vi "RG TAS v4b.vi"() -> ()   [LabVIEW 2015]
uses:
  <vilib>/Analysis/2dsp.llb/Decimate (single shot, DBL).vi
  <vilib>/DAQmx/read.llb/DAQmx Read (Analog Wfm 1Chan NSamp).vi
  Chaz TAS - DR/Sub VIs/Mono/global_Test.vi
  <vilib>/Instr/_visa.llb/VISA Configure Serial Port (Instr).vi
  Sub VIs/global tas.vi
  <vilib>/DAQmx/miscellaneous.llb/DAQmx Fill In Error Info.vi
  <vilib>/Utility/file.llb/Write To Spreadsheet File (DBL).vi
  <vilib>/Waveform/WDTOps.llb/WDT Index Channel DBL.vi
  Program Files/National Instruments/LabVIEW 2014/instr.lib/Tektronix DPO MSO 2000 4000 Series/Tektronix DPO MSO 2000 4000 Series.lvlib
  <vilib>/Analysis/NI_AALPro.lvlib
panel:
  in  "Inspect Traces":bool
  out "DAQ Loop":i32
  out "Scope Error Counter":i32
  out "Scope time axis":dbl[](array[numeric])
  in  "Stop acquisition":bool
  out "Grating":i32
  in  "2b - Spectrum":bool
  in  "2a - Kinetic":bool
  in  "Stop":bool
  out "Btrace Readout Counter":i32=2
  in  "Stop Btrace Measurement":bool
  out "Readout Counter":i32=2
  in  "Stop Measurement":bool
  in  "Calculate Output Method":T1(ring)
  in  "Parameters":T2(tab)
  in  "Shutter flow control":u16(ring) items=["None"=0, "XON/XOFF"=1, "RTS/CTS"=2, "DTR/DSR"=4]
  in  "Shutter stop bits":u16(ring)=10 items=["1.0"=10, "1.5"=15, "2.0"=20]
  in  "Shutter parity":u16(ring) items=["None", "Odd", "Even", "Mark", "Space"]
  in  "Shutter data bits":u16=8 min=5 max=8 step=1
  in  "Shutter VISA resource name":refnum<visa-resource-name>="COM1"
  in  "Shutter baud rate":u32=9600
  in  "Shutter open string":string="+100 10\n"
  in  "1 - Move Shutter":bool
  in  "3 - Move mono":bool
  out "Current wavelength (Oriel)":dbl format="%#_13g"
  in  "Monochromator Type":bool
  out "Start Wavelength":dbl min=0.0 format="%.3f"
  out "End Wavelength":dbl=100.0 min=0.0 format="%.3f"
  out "Interval Wavelength":dbl=10.0 min=0.0 format="%.3f"
  out "Current Wavelength (PTI)":dbl=300.0 min=300.0 max=2000.0 step=1.0
  in  "Is IR":bool caption="Grating"
  in  "Mono VISA name":refnum<visa-resource-name>
  in  "Mono 2 VISA name":refnum<visa-resource-name>
  out "DAQ dt":dbl=5e-06
  in  "DAQ End Time (s)":dbl=0.05
  in  "DAQ rate":i32=1250000
  in  "DAQ Trigger Level (V)":dbl=0.2
  out "DAQ Number of Samples":dbl=10000.0
  in  "DAQ average number of points":dbl=1.0
  out "DAQ final number of points":dbl
  in  "DAQ Input Channel":tag="Dev1/ai0"
  in  "100% Reflectance Standard (V)":dbl=1.0
  in  "DAQ Card":enum16{"USB-6211", "USB-6251"}(ring)=enum."USB-6251"
  in  "DAQ Input Config":i32(ring)=10106 items=["default"=-1, "RSE"=10083, "NRSE"=10078, "Differential"=10106, "Pseudodifferential"=12529]
  in  "Record Length":u32(ring)=10 items=["1000 points"=1, "10k points"=10, "100k points"=100, "1M points"=1000, "5M points"=5000, "10M points"=10000]
  in  "Acquisition Type":u16(ring)=2 items=["Sample", "Peak Detect", "Hi Res", "Envelope", "Average"]
  in  "Scope average\nnumber of points":dbl=1.0
  in  "Averages on scope":i32=1
  in  "Using TDS Scope?":bool
  in  "CH2 Impedance":u16(ring) items=["1M", "75", "50"]
  in  "CH1 Impedance":u16(ring)=2 items=["1M", "75", "50"]
  in  "Scope VISA resource name":refnum<visa-resource-name>="USB0::0x0699::0x0410::C022077::INSTR"
  in  "Scope Timeout (ms)":u32=30000
  in  "Channel TAS (0: Channel 1)":u16(ring) caption="Channel TAS" items=["Channel 1", "Channel 2", "Channel 3", "Channel 4", "Math", "Reference A", "Reference B", "Reference C", "Reference D"]
  in  "Channel TPC (0: Channel 1)":u16(ring)=1 caption="Channel TPC" items=["Channel 1", "Channel 2", "Channel 3", "Channel 4", "Math", "Reference A", "Reference B", "Reference C", "Reference D"]
  in  "Scope Timebase":dbl=0.0004 format="%^#_3e"
  in  "Trigger Source":u16(ring)=1 items=["Channel 1", "Channel 2", "Channel 3", "Channel 4", "AC Line", "Aux", "Digital Channel 0", "Digital Channel 1", "Digital Channel 2", "Digital Channel 3", "Digital Channel 4", "Digital Channel 5", "Digital Channel 6", "Digital Channel 7", "Digital Channel 8", "Digital Channel 9", "Digital Channel 10", "Digital Channel 11", "Digital Channel 12", "Digital Channel 13", "Digital Channel 14", "Digital Channel 15", "RF"]
  out "Final number of\nscope points":dbl=10000.0
  in  "Vertical Coupling TAS (1: DC)":u16(ring)=1 caption="Vertical Coupling TAS" items=["AC", "DC", "Ground"]
  in  "Probe Attenuation TAS (10.0)":dbl=1.0 caption="Probe Attenuation TAS"
  in  "Bandwidth CHTAS (0: FULL)":i32(ring) caption="Bandwidth CH TAS" items=["FULL", "250 MHz", "150 MHz", "20 MHz"]
  in  "Vertical Offset CH TAS (0.0 divs)":dbl=0.4 caption="Vertical Offset CH TAS (in V)"
  in  "Vertical Range CH TAS (10.0 V)":dbl=0.2 caption="Vertical Range CH TAS"
  in  "Trigger Level (V)":dbl=0.25
  in  "Vertical Coupling TPC (1: DC)":u16(ring)=1 caption="Vertical Coupling TPC" items=["AC", "DC", "Ground"]
  in  "Probe Attenuation TPC (1.0)":dbl=1.0 caption="Probe Attenuation TPC"
  in  "Vertical Range TPC (10.0 V)":dbl=0.2 caption="Vertical Range TPC"
  in  "Bandwidth CH TPC (0: FULL)":i32(ring) caption="Bandwidth CH TPC" items=["FULL", "250 MHz", "150 MHz", "20 MHz"]
  in  "Vertical Offset CH TPC (0.0 divs)":dbl caption="Vertical Offset CH TPC (in V)"
  in  "TPC Multiplication factor":dbl=1.0
  out "Number of scope readouts":i32
  in  "Scope Channel Read":bool
  in  "LED on (s)":dbl
  in  "LED off (s)":dbl
  in  "PIA Mode":bool
  in  "LEDs (constant irrad.)":bool caption="LEDs"
  in  "DAQ LED line":string="Dev1/port1/line0"
  in  "Control LEDs?":bool
  out "Scope pretrigger points":dbl=1000.0
  out "Scope CH1 DOD data (A-B final)":waveform(dbl)(graph)
  out "Scope CH1 DOD data (A final)":waveform(dbl)(graph)={"t0"=timestamp(-4.0000000000040004e-05 s since 1904-01-01), "dt"=4.0000000000000003e-07, "Y"=array[10000 elements]}
  out "Scope CH2 data (final)":waveform(dbl)(graph)={"t0"=timestamp(-4.0000000000040004e-05 s since 1904-01-01), "dt"=4.0000000000000003e-07, "Y"=array[10000 elements]}
  out "DAQ DOD data (final)":waveform(dbl)(graph)={"t0"=timestamp(0 s since 1904-01-01), "dt"=5e-06, "Y"=array[10000 elements]}
  out "B trace (Channel1)":waveform(dbl)(graph)
  in  "Amplification Factor":dbl=400.0
  out "Background level (on Amp)":dbl=30.577247161746392
  out "Background level (V)":dbl=0.08993307988748939
  in  "Trace B ?":bool
  out "Folder Created":bool
  in  "Sample Name":string="Sample"
  in  "TAS2014  Path":path=path "D:/Solar Fuels Data" caption="Folder"
  out "Path to Files":path=path "D:/Solar Fuels Data/Sample"
  out "Scope Average Channel2":waveform(dbl)(graph)={"t0"=timestamp(-4.0000000000040004e-05 s since 1904-01-01), "dt"=4.0000000000000003e-07, "Y"=array[10000 elements]}
  out "Scope Average Channel1":waveform(dbl)(graph)={"t0"=timestamp(-4.0000000000040004e-05 s since 1904-01-01), "dt"=4.0000000000000003e-07, "Y"=array[10000 elements]}
  out "DAQ Average Data":waveform(dbl)(graph)={"t0"=timestamp(0 s since 1904-01-01), "dt"=5e-06, "Y"=array[10000 elements]}
  in  "Number of Averages":i32=2
  out "DAQ Live Data":waveform(dbl)(graph)={"t0"=timestamp(0 s since 1904-01-01), "dt"=4.999999999999959e-06, "Y"=array[10000 elements]}
  # "Acquisition"
  # "Format: +100\\s20\\n OR \\F3\\002\\C1"
  # "Set COM ports for PTI\nmonochromators. If there\nis only 1 monochromator\npresent, leave Mono 2\nVISA name empty."
  # "DAQ Controls"
  # "DAQ Indicators"
  # "(Max = 250k/1.25M for\n6211/6251 DAQ cards)"
  # "Default is differential (connected ports are 15 and 16 on DAQ card).\n* For CH-TAS, input config should be RSE."
  # "Recommended Parameters for Different Scope Models"
  # "DPO3012"
  # "Record Length = 10k\nScope average number of points = 1"
  # "Acquisition Type = Hi Res\nAverages on scope = 1"
  # "DPO2012B"
  # "Record Length = 1M\nScope average number of points = 100"
  # "Acquisition Type = Average\nAverages on scope = 4"
  # "TDS3012C"
  # "Record Length = 10k\nScope average number of points = 1"
  # "Acquisition Type = Sample\nAverages on scope = 1"
  # "Channel 1"
  # "Channel 2"
  # "* For DPO2012B, impedance must be 1M for both channels!"
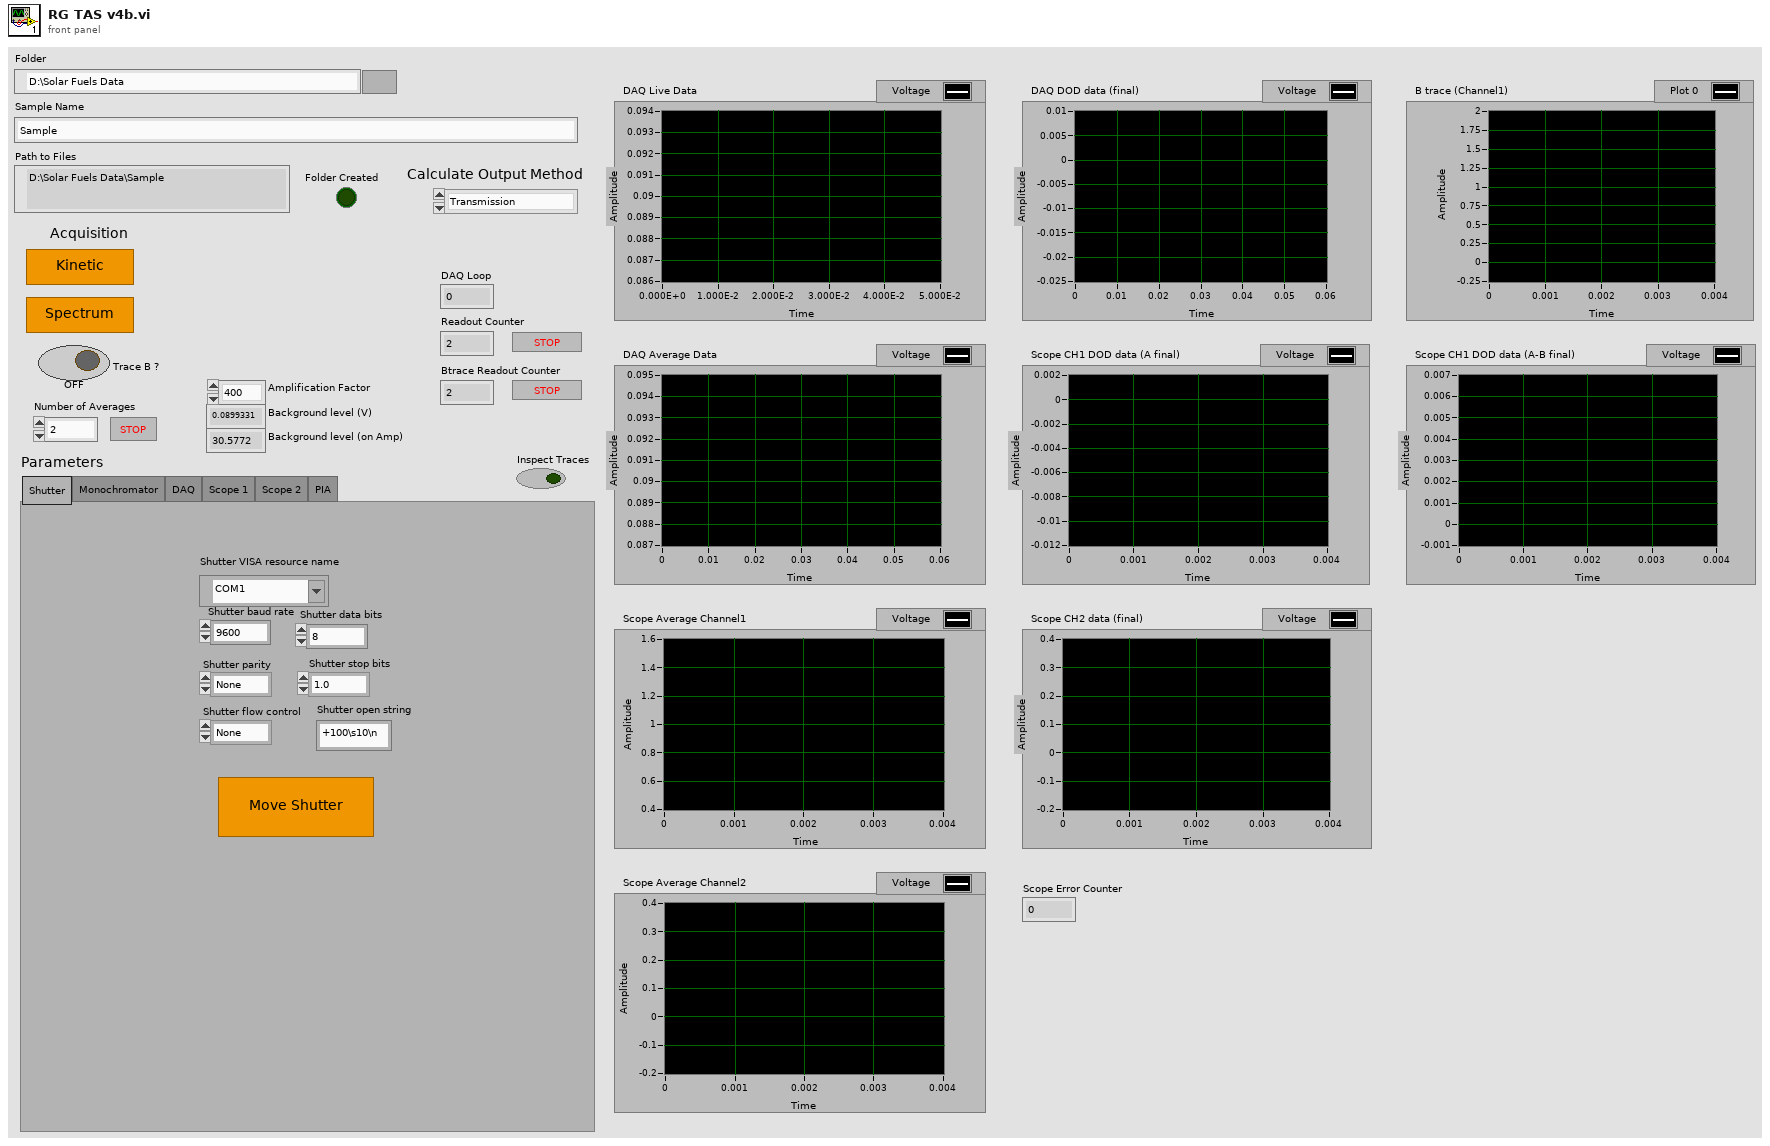
[diagram p1: front panel]
types:
  T1 = enum16{"Transmission", "Reflectance", "Kubelka-Munk"}
  T2 = enum32{"Shutter", "Monochromator", "DAQ", "Scope 1", "Scope 2", "PIA"}
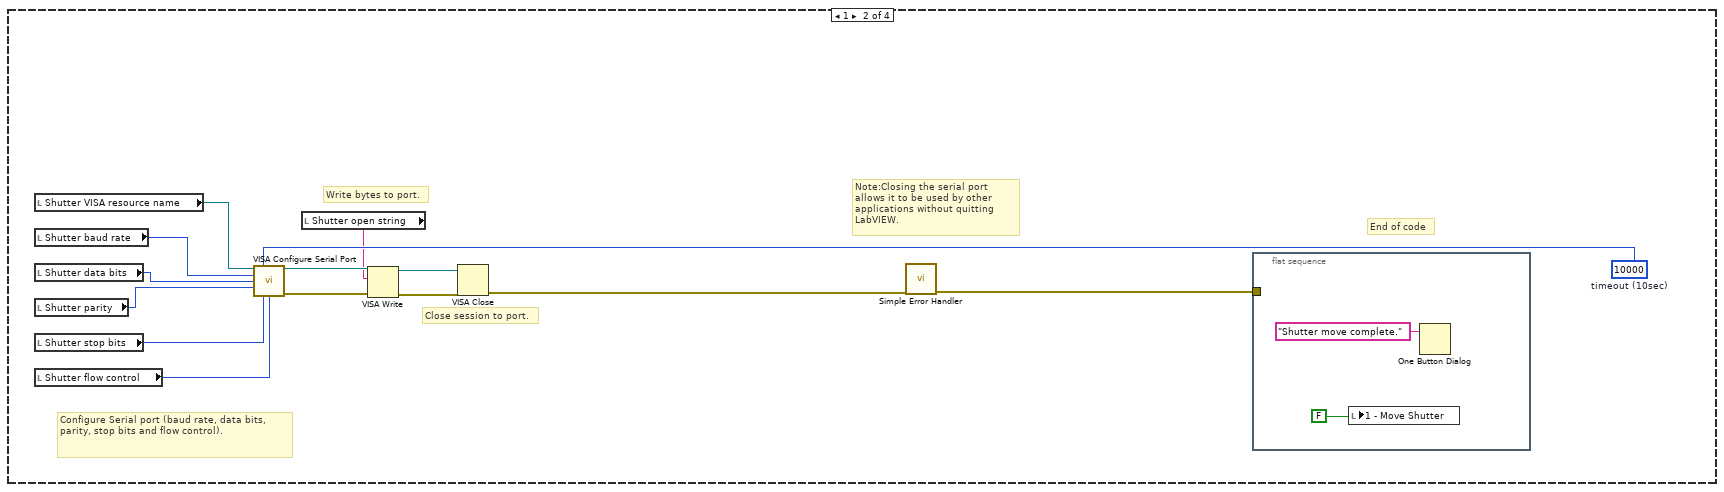
[diagram p4: hidden frame]
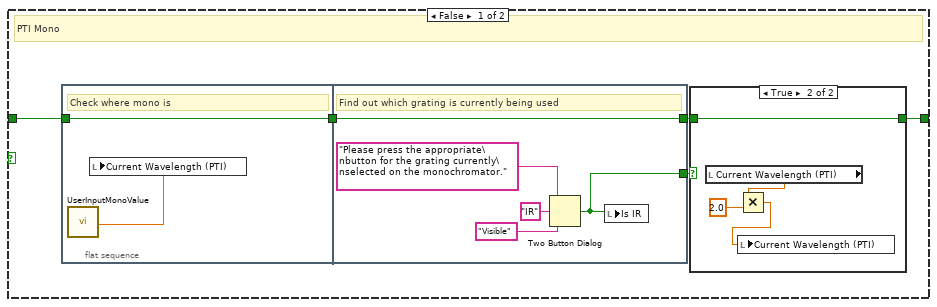
[diagram p5: hidden frame]
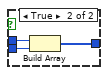
[diagram p8: hidden frame]
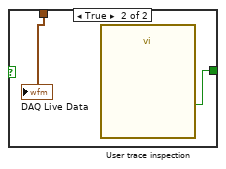
[diagram p9: hidden frame]
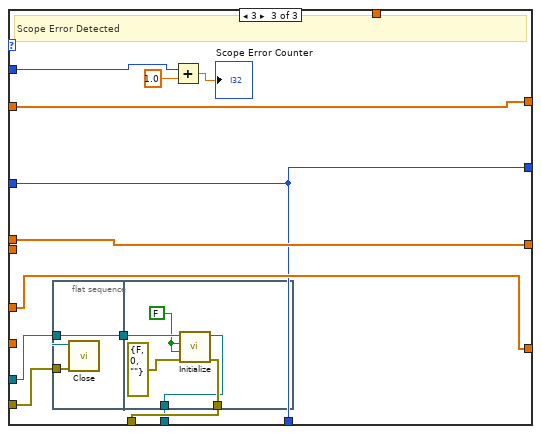
[diagram p11: hidden frame]
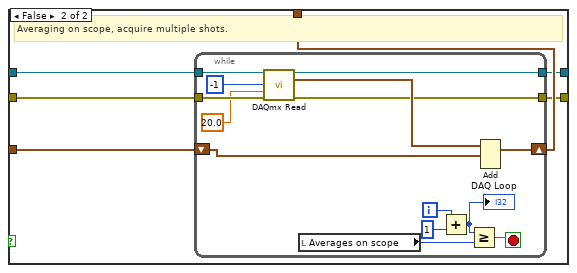
[diagram p13: hidden frame]
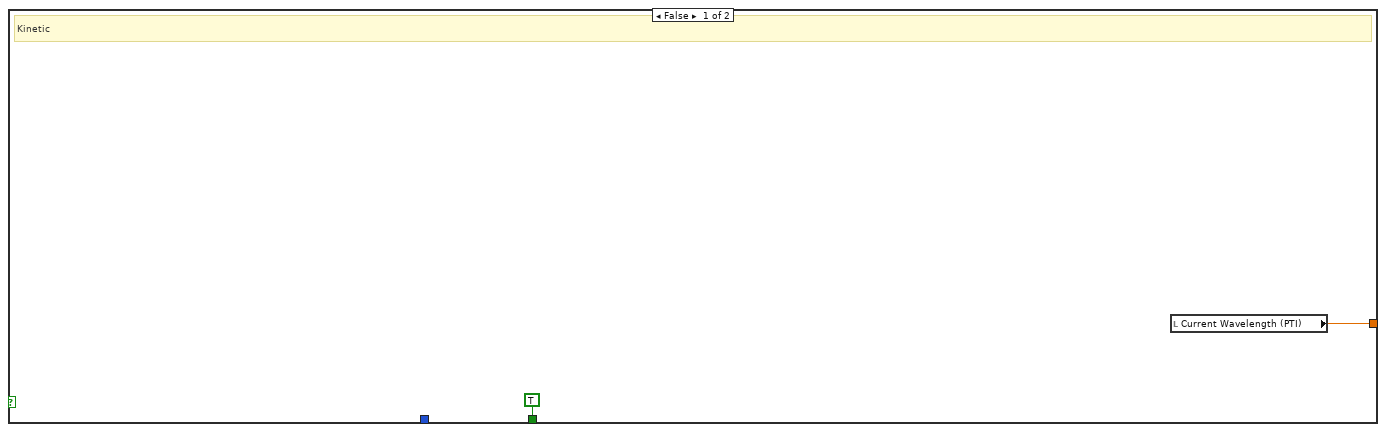
[diagram p14: hidden frame]
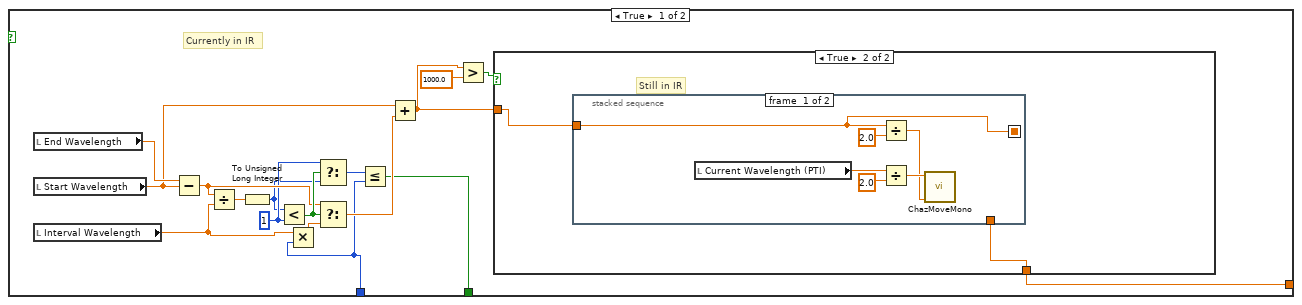
[diagram p15: hidden frame]
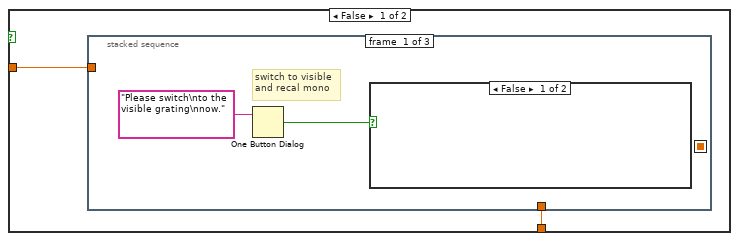
[diagram p16: hidden frame]
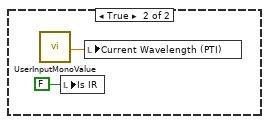
[diagram p17: hidden frame]
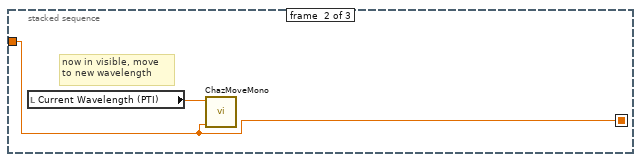
[diagram p18: hidden frame]
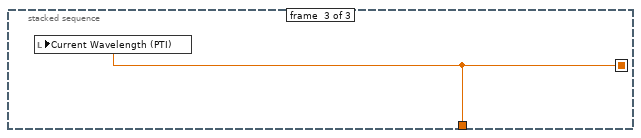
[diagram p19: hidden frame]
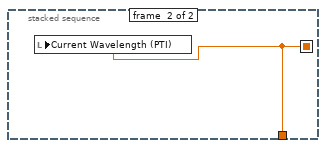
[diagram p20: hidden frame]
diagram:
  n1 = while {
    stop <- "Stop" stop-if-true
    # "True = Oriel"
    n2 = Or(x="2a - Kinetic", y="2b - Spectrum") -> (x .or. y?=w6:bool)
    n3 = Build Array(FALSE, "1 - Move Shutter", w6, "3 - Move mono") -> (w11:bool[])
    n4 = Search 1D Array(1D array=w11, element=TRUE) -> (index of element=w4:i32)  [unwired: 1 in]
    n5 = flat-sequence {
      tunnel: w4 -> [w37]
      tunnel: [w37] -> w3
      tunnel: "Monochromator Type" -> [w15]
      tunnel: [w15] -> w1
      frame #0 {
        # "Calculate DAQ parameters"
        # "Calculate Scope Parameters"
        n6 = case shown="True" "Control LEDs?" {
          frame False {
          }
          frame True {
            n7 = call "RG DAQ control for PIA.vi"("lines"="DAQ LED line", "Initial value"="LEDs (constant irrad.)") -> ()  [unwired: 10 in]
          }
        }
        n8 = Multiply(x="DAQ End Time (s)", y=1.1) -> (x*y=w16:dbl)
        n9 = Multiply(x="Record Length", y=u32 1000) -> (x*y=w25:u32)
        n10 = Multiply(x="DAQ rate", y=w16) -> (x*y=w24:dbl)
        "DAQ Number of Samples" <- w24
        n11 = Reciprocal(x="DAQ rate") -> (1/x=→"DAQ dt":dbl)
        n12 = Divide(x="Number of Averages", y="Averages on scope") -> (x/y=→"Number of scope readouts":dbl)
        n13 = Divide(x=w25, y="Scope average\nnumber of points") -> (x/y=w29:dbl)
        "Final number of\nscope points" <- w29
        n14 = Divide(x=w29, y=10.0) -> (x/y=→"Scope pretrigger points":dbl)
        n15 = Wait (ms)(milliseconds to wait=u32 1000) -> ()  [unwired: 1 out]
        n16 = Divide(x=w24, y="DAQ average number of points") -> (x/y=→"DAQ final number of points":dbl)
        n17 = global write "global_Test.vi" "Mono VISA name"("Mono VISA name") -> ()
        n18 = global write "global_Test.vi" "Mono 2 VISA name"("Mono 2 VISA name") -> ()
      }
    }
    n19 = case shown="2" w3 {
      tunnel: w1 -> [_ _ w56 w982]
      frame 0, Default {
      }
      frame 1 {
        w48 = u32 10000  # timeout (10sec)
        # "End of code"
        # "Note:Closing the serial port allows it to be used by other applications without quitting LabVIEW."
        # "Close session to port."
        # "Configure Serial port (baud rate, data bits, parity, stop bits and flow control)."
        # "Write bytes to port."
        n20 = local read "Shutter VISA resource name"() -> (w47:refnum<visa-resource-name>)
        n21 = local read "Shutter baud rate"() -> (w46:u32)
        n22 = local read "Shutter data bits"() -> (w45:u16)
        n23 = local read "Shutter parity"() -> (w44:u16)
        n24 = local read "Shutter stop bits"() -> (w43:u16)
        n25 = local read "Shutter flow control"() -> (w42:u16)
        n26 = call-poly "VISA Configure Serial Port"("VISA resource name"=w47, "timeout (10sec)"=w48, "baud rate (9600)"=w46, "data bits (8)"=w45, "parity (0:none)"=w44, "stop bits (10: 1 bit)"=w43, "flow control (0:none)"=w42) -> ("VISA resource name out"=w49:refnum<visa-resource-name>, "error out"=w50:errorcluster)  [unwired: 2 in, 5 out]
        n27 = local read "Shutter open string"() -> (w41:string)
        n28 = VISA Write(VISA resource name=w49, write buffer=w41, error in (no error)=w50) -> (VISA resource name out=w52:refnum<visa-resource-name>, error out=w53:errorcluster)  [unwired: 1 out]
        n29 = VISA Close(VISA resource name=w52, error in (no error)=w53) -> (error out=w51:errorcluster)
        n30 = call <vilib>:"Simple Error Handler.vi"("error in (no error)"=w51) -> ("error out"=w40:errorcluster)  [unwired: 1 in, 7 out]
        n31 = flat-sequence {
          tunnel: w40 -> [_]
          frame #0 {
            n32 = local write "1 - Move Shutter"(FALSE ("Move Shutter")) -> ()
            n33 = One Button Dialog(message="Shutter move complete.") -> ()  [unwired: 1 in, 1 out]
          }
        }
      }
      frame 2 {
        n34 = Build Path(base path="TAS2014  Path", name or relative path="Sample Name") -> (appended path=w67:path)
        n35 = call <vilib>:"Check if File or Folder Exists.vi"("path"=w67) -> ("file or folder exists?"=w66:bool, "dup path"=w65:path)  [unwired: 8 in, 1 out]
        n36 = case shown="True" w66 {
          tunnel: w65 -> [w974 w980]
          tunnel: [w973 w980] -> w60
          frame False {
            n37 = Create Folder(path (use dialog)=w974) -> (created path=w973:path)  [unwired: 2 in, 2 out]
            n38 = local write "Folder Created"(TRUE ("Folder Created")) -> ()
          }
          frame True {
            n39 = Two Button Dialog(message="Caution - folder already exists. Continue to overwrite data?", 1:"Yes, go for it!" ("F button name (\"Cancel\")"), 2:"No, help me!" ("T button name (\"OK\")")) -> (T button?=w975:bool)
            n40 = local write "Folder Created"(FALSE ("Folder Created")) -> ()
            n41 = Stop(stop? (T)=w975) -> ()
          }
        }
        "Path to Files" <- w60
        n42 = case shown="True" w56 {
          tunnel: w56 -> [w71 w86]
          tunnel: [w69 w85] -> w57
          frame False {
            # "PTI Mono"
            n43 = flat-sequence {
              tunnel: [w78] -> w72
              tunnel: w71 -> [w78]
              tunnel: w72 -> [w84]
              tunnel: [w84] -> w70
              tunnel: [w80] -> w68
              frame #0 {
                # "Check where mono is"
                n44 = call "UserInputMonoValue.vi"() -> ("Monochromator readout"=w79:dbl)  [unwired: 17 in, 2 out]
                n45 = local write "Current Wavelength (PTI)"(w79) -> ()
              }
              frame #1 {
                # "Find out which grating is currently being used"
                n46 = Two Button Dialog(message="Please press the appropriate\nbutton for the grating currently\nselected on the monochromator.", 1:"Visible" ("F button name (\"Cancel\")"), 2:"IR" ("T button name (\"OK\")")) -> (T button?=w80:bool)
                n47 = local write "Is IR"(w80) -> ()
              }
            }
            n48 = case shown="True" w68 {
              tunnel: w70 -> [w73 w77]
              tunnel: [w73 w77] -> w69
              frame False {
              }
              frame True {
                n49 = local read "Current Wavelength (PTI)"() -> (w75:dbl)
                n50 = Multiply(x=w75, y=2.0) -> (x*y=w74:dbl)
                n51 = local write "Current Wavelength (PTI)"(w74) -> ()
              }
            }
          }
          frame True {
            # "Oriel Mono"
            n52 = flat-sequence {
              tunnel: w86 -> [w90]
              tunnel: [w90] -> w85
              frame #0 {
                n53 = call "m_open.vi"() -> ("error out"=w91:errorcluster, "configuration file path copy"=w87:path)  [unwired: 2 in]
                n54 = call "GetWave.vi"("error in (no error)"=w91) -> ("error out"=w89:errorcluster, "Present Wavelength"=w88:dbl)  [unwired: 1 in]
                n55 = call "m_close.vi"("error in (no error)"=w89, "configuration file path"=w87) -> ()  [unwired: 2 out]
                n56 = local write "Current wavelength (Oriel)"(w88) -> ()
              }
            }
          }
        }
        n57 = local read "2b - Spectrum"() -> (w62:bool)
        n58 = global write "global tas.vi" "Root Path"(w60) -> ()
        n59 = case shown="True" w62 {
          tunnel: w60 -> [w95 w96]
          tunnel: [w95 w96] -> w58
          frame False {
          }
          frame True {
            n60 = call "RG Get Spectrum Wavelengths.vi"() -> ("Wavelength interval"=→"Interval Wavelength":i32, "End wavelength"=→"End Wavelength":i32, "Start wavelength"=→"Start Wavelength":i32)  [unwired: 9 in]
          }
        }
        n61 = flat-sequence {
          tunnel: [w92] -> w59
          tunnel: w58 -> [_]
          frame #0 {
            n62 = call "Prompt User for Input"() -> ("yes"=w92:bool)  [unwired: 18 in, 1 out]
          }
        }
        n63 = while {
          tunnel: [w177] -> w61
          tunnel: w59 -> [w172]
          tunnel: w57 -> [w165]
          i -> [w166]
          stop <- w196 stop-if-true
          w257 = TRUE  # Reset (True)
          w131 = 0
          w260 = FALSE  # ID Query (True)
          w293 = FALSE  # Enable Continuous Acquisition Mode (True)
          # "Scope t0"
          # "Scope dt"
          # "DAQ index to make\nsure DAQ acquisition\nis finished before\ndoing B trace."
          # "Scope time\naxis"
          # "Scope time axis"
          # "Current wavelength"
          # "Current Wavelength"
          # "Make sure the 20s is waited before starting to acquire the data if shutter moves."
          # "Set time so that trigger\nis at t = 0"
          # "Get pre laser light level"
          # "Change cases for old TDS scope models because of differences in programming commands."
          # "Get pre laser light level (V) for DAQ and Scope"
          # "Disable time delay"
          # "Configure Timebase"
          # "Disable continous acquisition"
          # "Configure Trigger"
          # "If reading 2 channels, combine Channel A\n and Channel B so that both channels are read"
          # "Configure Channel B"
          # "Configure Channel A"
          # "Check the initial position of the shutter, and move if Doing Trace B and Spectrum"
          n64 = local read "2b - Spectrum"() -> (w169:bool)
          n65 = case shown="False" w165 {
            tunnel: [w534 w625] -> w195
            tunnel: [w531 w624] -> w193
            tunnel: [w533 w623] -> w176
            tunnel: w169 -> [w535 w622]
            tunnel: w166 -> [w536 w621]
            frame False {
              # "PTI Monochromator"
              n66 = flat-sequence {
                tunnel: w536 -> [w540]
                tunnel: w535 -> [w539]
                tunnel: [w538] -> w534
                tunnel: [w537] -> w532
                tunnel: [w620] -> w533
                tunnel: w532 -> [w620]
                tunnel: [w619] -> w531
                frame #0 {
                  n67 = case shown="True" w539 {
                    tunnel: w540 -> [_ w545]
                    tunnel: [TRUE w544] -> w538
                    tunnel: [w542 w543] -> w537
                    frame False {
                      # "Kinetic"
                      n68 = local read "Current Wavelength (PTI)"() -> (w542:dbl)
                    }
                    frame True {
                      # "Spectrum"
                      n69 = case shown="False" "Is IR" {
                        tunnel: w545 -> [w549 w585]
                        tunnel: [w550 w584] -> w544
                        tunnel: [w548 w583] -> w543
                        frame True {
                          w558 = u32 1 ("y")
                          # "Currently in IR"
                          n70 = local read "End Wavelength"() -> (w556:dbl)
                          n71 = local read "Start Wavelength"() -> (w554:dbl)
                          n72 = local read "Interval Wavelength"() -> (w551:dbl)
                          n73 = Subtract(x=w556, y=w554) -> (x-y=w559:dbl)
                          n74 = Divide(x=w559, y=w551) -> (x/y=w561:dbl)
                          n75 = To Unsigned Long Integer(number=w561) -> (unsigned 32bit integer=w557:u32)
                          n76 = Less?(x=w557, y=w558) -> (x < y?=w560:bool)
                          n77 = Multiply(x=w551, y=w549) -> (x*y=w552:dbl)
                          n78 = Select(t=w558, s=w560, f=w557) -> (s? t:f=w555:u32)
                          n79 = Select(t=w559, s=w560, f=w552) -> (s? t:f=w553:dbl)
                          n80 = Less Or Equal?(x=w555, y=w549) -> (x <= y?=w550:bool)
                          n81 = Add(x=w554, y=w553) -> (x+y=w547:dbl)
                          n82 = Greater?(x=w547, y=1000.0) -> (0:w562:bool)
                          n83 = case shown="True" w562 {
                            tunnel: [w565 w574] -> w548
                            tunnel: w547 -> [w564 w573]
                            frame False {
                              n84 = stacked-sequence {
                                seq-local: [_ w570 _] -> [_ _ w572]
                                tunnel: [_ _ w572] -> w565
                                tunnel: w564 -> [_ w570 _]
                                frame #0 {
                                # "switch to visible\nand recal mono"
                                n85 = One Button Dialog(message="Please switch\nto the visible grating\nnow.") -> (true=w566:bool)  [unwired: 1 in]
                                n86 = case shown="False" w566 {
                                frame False {
                                }
                                frame True {
                                n87 = call "UserInputMonoValue.vi"() -> ("Monochromator readout"=w568:dbl)  [unwired: 17 in, 2 out]
                                n88 = local write "Is IR"(FALSE ("Is IR")) -> ()
                                n89 = local write "Current Wavelength (PTI)"(w568) -> ()
                                }
                                }
                                }
                                frame #1 {
                                # "now in visible, move \nto new wavelength"
                                n90 = local read "Current Wavelength (PTI)"() -> (w571:dbl)
                                n91 = call "ChazMoveMono.vi"("Move to"=w570, "Current"=w571) -> ()  [unwired: 8 in, 2 out]
                                }
                                frame #2 {
                                n92 = local write "Current Wavelength (PTI)"(w572) -> ()
                                }
                              }
                            }
                            frame True {
                              # "Still in IR"
                              n93 = stacked-sequence {
                                seq-local: [w575 _] -> [_ w581]
                                tunnel: [_ w581] -> w574
                                tunnel: w573 -> [w575 _]
                                frame #0 {
                                n94 = local read "Current Wavelength (PTI)"() -> (w580:dbl)
                                n95 = Divide(x=w575, y=2.0) -> (x/y=w576:dbl)
                                n96 = Divide(x=w580, y=2.0) -> (x/y=w577:dbl)
                                n97 = call "ChazMoveMono.vi"("Move to"=w576, "Current"=w577) -> ()  [unwired: 8 in, 2 out]
                                }
                                frame #1 {
                                n98 = local write "Current Wavelength (PTI)"(w581) -> ()
                                }
                              }
                            }
                          }
                        }
                        frame False {
                          w593 = u32 1 ("y")
                          # "Currently in Visible"
                          n99 = local read "End Wavelength"() -> (w591:dbl)
                          n100 = local read "Start Wavelength"() -> (w589:dbl)
                          n101 = local read "Interval Wavelength"() -> (w586:dbl)
                          n102 = Subtract(x=w591, y=w589) -> (x-y=w594:dbl)
                          n103 = Divide(x=w594, y=w586) -> (x/y=w596:dbl)
                          n104 = To Unsigned Long Integer(number=w596) -> (unsigned 32bit integer=w592:u32)
                          n105 = Less?(x=w592, y=w593) -> (x < y?=w595:bool)
                          n106 = Multiply(x=w586, y=w585) -> (x*y=w587:dbl)
                          n107 = Select(t=w593, s=w595, f=w592) -> (s? t:f=w590:u32)
                          n108 = Select(t=w594, s=w595, f=w587) -> (s? t:f=w588:dbl)
                          n109 = Less Or Equal?(x=w590, y=w585) -> (x <= y?=w584:bool)
                          n110 = Add(x=w589, y=w588) -> (x+y=w582:dbl)
                          n111 = Greater?(x=w582, y=1000.0) -> (0:w597:bool)
                          n112 = case shown="False" w597 {
                            tunnel: [w600 w605] -> w583
                            tunnel: w582 -> [w599 w604]
                            frame False {
                              # "Still in Visible"
                              n113 = stacked-sequence {
                                seq-local: [w601 _] -> [_ w603]
                                tunnel: [_ w603] -> w600
                                tunnel: w599 -> [w601 _]
                                frame #0 {
                                n114 = local read "Current Wavelength (PTI)"() -> (w602:dbl)
                                n115 = call "ChazMoveMono.vi"("Move to"=w601, "Current"=w602) -> ()  [unwired: 8 in, 2 out]
                                }
                                frame #1 {
                                n116 = local write "Current Wavelength (PTI)"(w603) -> ()
                                }
                              }
                            }
                            frame True {
                              n117 = stacked-sequence {
                                seq-local: [_ w612 _] -> [_ _ w618]
                                tunnel: [_ _ w618] -> w605
                                tunnel: w604 -> [_ w612 _]
                                frame #0 {
                                # "switch to IR\nand recal mono"
                                n118 = One Button Dialog(message="Please switch\nto the IR grating\nnow.") -> (true=w606:bool)  [unwired: 1 in]
                                n119 = case shown="True" w606 {
                                frame False {
                                }
                                frame True {
                                n120 = call "UserInputMonoValue.vi"() -> ("Monochromator readout"=w610:dbl)  [unwired: 17 in, 2 out]
                                n121 = local write "Is IR"(TRUE ("Is IR")) -> ()
                                n122 = Multiply(x=w610, y=2.0) -> (x*y=w608:dbl)
                                n123 = local write "Current Wavelength (PTI)"(w608) -> ()
                                }
                                }
                                }
                                frame #1 {
                                # "now in IR, move \nto new wavelength"
                                n124 = local read "Current Wavelength (PTI)"() -> (w615:dbl)
                                n125 = Divide(x=w612, y=2.0) -> (x/y=w613:dbl)
                                n126 = Divide(x=w615, y=2.0) -> (x/y=w614:dbl)
                                n127 = call "ChazMoveMono.vi"("Move to"=w613, "Current"=w614) -> ()  [unwired: 8 in, 2 out]
                                }
                                frame #2 {
                                n128 = local write "Current Wavelength (PTI)"(w618) -> ()
                                }
                              }
                            }
                          }
                        }
                      }
                    }
                  }
                }
                frame #1 {
                  n129 = call <vilib>:"General Error Handler.vi"() -> ("error out"=w619:errorcluster)  [unwired: 11 in, 4 out]
                }
              }
            }
            frame True {
              # "Oriel Monochromator"
              n130 = case shown="False" w622 {
                tunnel: [TRUE w655] -> w625
                tunnel: w621 -> [_ w642]
                tunnel: [w627 w640] -> w624
                tunnel: [w626 w639] -> w623
                frame False {
                  # "B trace OFF"
                  n131 = call "m_open.vi"() -> ("error out"=w629:errorcluster, "configuration file path copy"=w628:path)  [unwired: 2 in]
                  n132 = call "GetWave.vi"("error in (no error)"=w629) -> ("error out"=w637:errorcluster, "Present Wavelength"=w626:dbl)  [unwired: 1 in]
                  "Current wavelength (Oriel)" <- w626
                  n133 = Less Or Equal?(x=w626, y=590.0) -> (x <= y?=w636:bool)
                  n134 = Select(t=1.0, s=w636, f=2.0) -> (s? t:f=w633:dbl)
                  n135 = call "setgrat.vi"("error in (no error)"=w637, "Grating"=w633) -> ("error out"=w634:errorcluster)  [unwired: 1 in]
                  n136 = call "gowave.vi"("error in (no error)"=w634, "Destination Wavelength"=w626) -> ("error out"=w635:errorcluster)
                  n137 = call "m_close.vi"("error in (no error)"=w635, "configuration file path"=w628) -> ("error out"=w627:errorcluster)  [unwired: 1 out]
                }
                frame True {
                  w659 = u32 1 ("y")
                  # "B trace ON"
                  n138 = local read "End Wavelength"() -> (w657:dbl)
                  n139 = local read "Start Wavelength"() -> (w646:dbl)
                  n140 = local read "Interval Wavelength"() -> (w643:dbl)
                  n141 = Subtract(x=w657, y=w646) -> (x-y=w660:dbl)
                  n142 = Divide(x=w660, y=w643) -> (x/y=w662:dbl)
                  n143 = To Unsigned Long Integer(number=w662) -> (unsigned 32bit integer=w658:u32)
                  n144 = Less?(x=w658, y=w659) -> (x < y?=w661:bool)
                  n145 = Multiply(x=w643, y=w642) -> (x*y=w644:dbl)
                  n146 = Select(t=w659, s=w661, f=w658) -> (s? t:f=w656:u32)
                  n147 = Select(t=w660, s=w661, f=w644) -> (s? t:f=w645:dbl)
                  n148 = Less Or Equal?(x=w656, y=w642) -> (x <= y?=w655:bool)
                  n149 = Add(x=w646, y=w645) -> (x+y=w639:dbl)
                  n150 = call "m_open.vi"() -> ("error out"=w641:errorcluster, "configuration file path copy"=w654:path)  [unwired: 2 in]
                  n151 = Less Or Equal?(x=w639, y=590.0) -> (x <= y?=w647:bool)
                  n152 = local write "Current wavelength (Oriel)"(w639) -> ()
                  n153 = Select(t=1.0, s=w647, f=2.0) -> (s? t:f=w650:dbl)
                  n154 = call "setgrat.vi"("error in (no error)"=w641, "Grating"=w650) -> ("error out"=w649:errorcluster)  [unwired: 1 in]
                  n155 = call "gowave.vi"("error in (no error)"=w649, "Destination Wavelength"=w639) -> ("error out"=w648:errorcluster)
                  n156 = call "m_close.vi"("error in (no error)"=w648, "configuration file path"=w654) -> ("error out"=w640:errorcluster)  [unwired: 1 out]
                }
              }
            }
          }
          n157 = local read "Scope VISA resource name"() -> (w303:refnum<visa-resource-name>)
          n158 = local read "Trace B ?"() -> (w170:bool)
          n159 = And(x=w170, y=w169) -> (x .and. y?=w168:bool)
          n160 = Not Equal To 0?(x=w166) -> (x != 0?=w167:bool)
          n161 = And(x=w168, y=w167) -> (x .and. y?=w171:bool)
          n162 = Or(x=w172, y=w171) -> (x .or. y?=w173:bool)
          n163 = call "Initialize.vi"("error in (no error)"=w193, "Reset (True)"=w257, "ID Query (True)"=w260, "VISA resource name"=w303) -> ("error out"=w295:errorcluster, "VISA resource name out"=w294:refnum<visa-resource-name>)  [unwired: 6 in]
          n164 = local read "Scope Timeout (ms)"() -> (w125:u32)
          n165 = case shown="True" w173 {
            tunnel: [u32 0 ("millisecond timer value") w957] -> w110
            frame False {
            }
            frame True {
              w967 = u32 10000  # timeout (10sec)
              # "Note:Closing the serial port allows it to be used by other applications without quitting LabVIEW."
              # "Close session to port."
              # "Configure Serial port (baud rate, data bits, parity, stop bits and flow control)."
              # "Write bytes to port."
              n166 = call-poly "VISA Configure Serial Port"("VISA resource name"="Shutter VISA resource name", "timeout (10sec)"=w967, "baud rate (9600)"="Shutter baud rate", "data bits (8)"="Shutter data bits", "parity (0:none)"="Shutter parity", "stop bits (10: 1 bit)"="Shutter stop bits", "flow control (0:none)"="Shutter flow control") -> ("VISA resource name out"=w963:refnum<visa-resource-name>, "error out"=w962:errorcluster)  [unwired: 2 in, 5 out]
              n167 = VISA Write(VISA resource name=w963, write buffer="Shutter open string", error in (no error)=w962) -> (VISA resource name out=w960:refnum<visa-resource-name>, error out=w959:errorcluster)  [unwired: 1 out]
              n168 = VISA Close(VISA resource name=w960, error in (no error)=w959) -> (error out=w961:errorcluster)
              n169 = call <vilib>:"Simple Error Handler.vi"("error in (no error)"=w961) -> ()  [unwired: 1 in, 8 out]
              n170 = Wait (ms)(milliseconds to wait=u32 20000) -> (millisecond timer value=w957:u32)
            }
          }
          n171 = call "Configure Continuous Acquisition.vi"("error in (no error)"=w295, "Enable Continuous Acquisition Mode (T: Enable)"=w293, "VISA resource name"=w294) -> ("error out"=w129:errorcluster, "VISA resource name out"=w130:refnum<visa-resource-name>)  [unwired: 7 in]
          n172 = local read "Vertical Range CH TAS (10.0 V)"() -> (w288:dbl)
          n173 = local read "Vertical Offset CH TAS (0.0 divs)"() -> (w305:dbl)
          n174 = property class="Instr"(reference=w130, error in=w129, "General Settings:Timeout Value"=w125) -> (reference out=w128:refnum<visa-resource-name>, error out=w127:errorcluster)
          n175 = local read "Vertical Coupling TAS (1: DC)"() -> (w286:u16)
          n176 = local read "Bandwidth CHTAS (0: FULL)"() -> (w284:i32)
          n177 = local read "Probe Attenuation TAS (10.0)"() -> (w304:dbl)
          n178 = local read "Channel TAS (0: Channel 1)"() -> (w285:u16)
          n179 = Or(x=w195, y="Stop acquisition") -> (x .or. y?=w196:bool)
          n180 = local read "Vertical Offset CH TPC (0.0 divs)"() -> (w302:dbl)
          n181 = local read "Vertical Coupling TPC (1: DC)"() -> (w282:u16)
          n182 = local read "Probe Attenuation TPC (1.0)"() -> (w301:dbl)
          n183 = local read "Channel TPC (0: Channel 1)"() -> (w283:u16)
          n184 = local read "Vertical Range TPC (10.0 V)"() -> (w287:dbl)
          n185 = local read "Bandwidth CH TPC (0: FULL)"() -> (w281:i32)
          n186 = local read "Scope Timebase"() -> (w108:dbl)
          n187 = local read "Record Length"() -> (w278:u32)
          n188 = case shown="False" "Using TDS Scope?" {
            tunnel: w305 -> [w927 w955]
            tunnel: w304 -> [w926 w954]
            tunnel: w302 -> [w925 w953]
            tunnel: w301 -> [w924 w952]
            tunnel: w127 -> [w923 w951]
            tunnel: w128 -> [w922 w950]
            tunnel: w288 -> [w919 w947]
            tunnel: w287 -> [w918 w946]
            tunnel: w286 -> [w915 w943]
            tunnel: w285 -> [w914 w942]
            tunnel: w284 -> [w913 w941]
            tunnel: w283 -> [w912 w940]
            tunnel: w282 -> [w911 w939]
            tunnel: w281 -> [w910 w938]
            tunnel: w278 -> [w909 w937]
            tunnel: [w907 w935] -> w277
            tunnel: [w905 w933] -> w276
            tunnel: "CH1 Impedance" -> [w903 w931]
            tunnel: "CH2 Impedance" -> [w902 w930]
            tunnel: w108 -> [w901 w929]
            tunnel: 10.0 ("Position (10 %)") -> [w900 w928]
            frame True {
              n189 = call "RG Configure Channel TDS3012C.vi"("VISA resource name"=w922, "Input Impedance (0: 1M ohm)"=w903, "Channel (0: Channel 1)"=w914, "Vertical Coupling (1: DC)"=w915, "Probe Attenuation (1)"=w926, "error in (no error)"=w923, "Vertical Range (10.0 V)"=w919, "Vertical Offset (0.0 V)"=w927, "Bandwidth (0: FULL)"=w913) -> ("VISA resource name out"=w921:refnum<visa-resource-name>, "error out"=w920:errorcluster)  [unwired: 5 in]
              n190 = call "RG Configure Channel TDS3012C.vi"("VISA resource name"=w921, "Input Impedance (0: 1M ohm)"=w902, "Channel (0: Channel 1)"=w912, "Vertical Coupling (1: DC)"=w911, "Probe Attenuation (1)"=w924, "error in (no error)"=w920, "Vertical Range (10.0 V)"=w918, "Vertical Offset (0.0 V)"=w925, "Bandwidth (0: FULL)"=w910) -> ("VISA resource name out"=w916:refnum<visa-resource-name>, "error out"=w917:errorcluster)  [unwired: 5 in]
              n191 = call "RG Configure Timebase TDS3012C.vi"("Record Length (10: 10k points)"=w909, "error in (no error)"=w917, "Position (10 %)"=w900, "Timebase (0.0005 s)"=w901, "VISA resource name"=w916) -> ("error out"=w906:errorcluster, "VISA resource name out"=w908:refnum<visa-resource-name>)  [unwired: 5 in]
              n192 = call "RG Configure Delay TDS3012C.vi"("error in (no error)"=w906, "Enable Delay (T: Enable)"=FALSE, "VISA resource name"=w908) -> ("error out"=w905:errorcluster, "VISA resource name out"=w907:refnum<visa-resource-name>)  [unwired: 7 in]
            }
            frame False {
              n193 = call "Configure Channel.vi"("VISA resource name"=w950, "Input Impedance (0: 1M ohm)"=w931, "Channel (0: Channel 1)"=w942, "Vertical Coupling (1: DC)"=w943, "Probe Attenuation (1)"=w954, "error in (no error)"=w951, "Vertical Range (10.0 V)"=w947, "Vertical Offset (0.0 V)"=w955, "Bandwidth (0: FULL)"=w941) -> ("VISA resource name out"=w949:refnum<visa-resource-name>, "error out"=w948:errorcluster)  [unwired: 5 in]
              n194 = call "Configure Channel.vi"("VISA resource name"=w949, "Input Impedance (0: 1M ohm)"=w930, "Channel (0: Channel 1)"=w940, "Vertical Coupling (1: DC)"=w939, "Probe Attenuation (1)"=w952, "error in (no error)"=w948, "Vertical Range (10.0 V)"=w946, "Vertical Offset (0.0 V)"=w953, "Bandwidth (0: FULL)"=w938) -> ("VISA resource name out"=w944:refnum<visa-resource-name>, "error out"=w945:errorcluster)  [unwired: 5 in]
              n195 = call "Configure Timebase.vi"("Record Length (10: 10k points)"=w937, "error in (no error)"=w945, "Position (10 %)"=w928, "Timebase (0.0005 s)"=w929, "VISA resource name"=w944) -> ("error out"=w934:errorcluster, "VISA resource name out"=w936:refnum<visa-resource-name>)  [unwired: 5 in]
              n196 = call "Configure Delay.vi"("error in (no error)"=w934, "Enable Delay (T: Enable)"=FALSE, "VISA resource name"=w936) -> ("error out"=w933:errorcluster, "VISA resource name out"=w935:refnum<visa-resource-name>)  [unwired: 7 in]
            }
          }
          n197 = Multiply(x=w108, y=1800.0) -> (x*y=w106:dbl)
          n198 = flat-sequence {
            tunnel: [w313] -> w124
            tunnel: [w312] -> w123
            tunnel: [w311] -> w117
            tunnel: w110 -> [w310]
            tunnel: [w310] -> w109
            frame #0 {
              # "DAQ Setup acquisition"
              n199 = local read "DAQ Number of Samples"() -> (w314:dbl)
              n200 = local read "DAQ Trigger Level (V)"() -> (w321:dbl)
              n201 = local read "DAQ Input Channel"() -> (w322:tag)
              n202 = local read "DAQ rate"() -> (w315:i32)
              n203 = call "RG Configure DAQ auto Max input scale.vi"("input terminal configuration"="DAQ Input Config", "DAQ Card Type"="DAQ Card", "Sampling rate"=w315, "DAQ Trigger Level"=w321, "physical channel"=w322, "number of samples"=w314) -> ("error out"=w313:errorcluster, "task out"=w312:refnum<k21>)  [unwired: 4 in]
              n204 = Reciprocal(x=w315) -> (1/x=w316:dbl)
              n205 = Initialize Array(0.0 ("element"), w314) -> (w317:dbl[])
              n206 = Bundle By Name("Y"=w317, "dt"=w316) -> (w311:waveform(dbl))  [unwired: 1 in]
            }
          }
          n207 = Max & Min(x=w106, y=700.0) -> (max(x,y)=w104:dbl)  [unwired: 1 out]
          n208 = local read "Trigger Level (V)"() -> (w280:dbl)
          n209 = local read "Trigger Source"() -> (w279:u16)
          n210 = local read "DAQ final number of points"() -> (w136:dbl)
          n211 = case shown="False" "Scope Channel Read" {
            tunnel: [w323 w327] -> w296
            tunnel: w285 -> [w324 w326]
            tunnel: w283 -> [_ w325]
            frame False {
              n212 = Build Array(w324) -> (w323:u16[])
            }
            frame True {
              n213 = Build Array(w326, w325) -> (w327:u16[])
            }
          }
          n214 = local read "Averages on scope"() -> (w201:i32)
          n215 = call "RG Configure Trigger (Edge).vi"("VISA resource name"=w277, "Trigger Source (0: Channel 1)"=w279, "Trigger Level (0.0 V)"=w280, "error in (no error)"=w276) -> ("VISA resource name out"=w272:refnum<visa-resource-name>, "error out"=w273:errorcluster)  [unwired: 10 in]
          n216 = local read "Final number of\nscope points"() -> (w266:dbl)
          n217 = call "Configure Acquisition.vi"("error in (no error)"=w273, "Number of Waveform Acquisitions (16)"=w201, "Acquisition Type (0: Sample)"="Acquisition Type", "VISA resource name"=w272) -> ("error out"=w101:errorcluster, "VISA resource name out"=w103:refnum<visa-resource-name>)  [unwired: 6 in]
          n218 = local write "Scope Error Counter"(w131) -> ()
          n219 = flat-sequence {
            tunnel: w103 -> [w309]
            tunnel: [w309] -> w102
            tunnel: w101 -> [w308]
            tunnel: [w308] -> w100
            frame #0 {
              n220 = Wait (ms)(milliseconds to wait=u32 1000) -> ()  [unwired: 1 out]
            }
          }
          n221 = Initialize Array(0.0 ("element"), w136) -> (w134:dbl[])
          n222 = Initialize Array(0.0 ("element"), w266) -> (w133:dbl[])
          n223 = while {
            tunnel: w296 -> [w352]
            tunnel: [w351] -> w163
            shift-right: [w362] -> w142
            shift-left: w100 -> [w356]
            shift-right: [w358] -> w143
            shift-left: w102 -> [w357]
            shift-right: [w387] -> w263
            shift-left: w133 -> [w370]
            shift-right: [w388] -> w297
            shift-left: w134 -> [w368]
            shift-right: [w364] -> w119
            shift-left: w131 -> [w369]
            shift-right: [w366] -> w264
            shift-left: w133 -> [w365]
            tunnel: 0 -> [w363]
            tunnel: w124 -> [w347]
            tunnel: w123 -> [w348]
            tunnel: [w346] -> w122
            tunnel: [w345] -> w121
            tunnel: w117 -> [w344]
            tunnel: w109 -> [_]
            tunnel: w104 -> [w336]
            stop <- w371 stop-if-true
            w328 = TRUE ("element")
            n224 = flat-sequence {
              tunnel: w357 -> [w454]
              tunnel: [w451] -> w353
              tunnel: [w450] -> w354
              tunnel: [w458] -> w343
              tunnel: w356 -> [w453]
              tunnel: w348 -> [w449]
              tunnel: w347 -> [w448]
              tunnel: [w447] -> w346
              tunnel: [w446] -> w345
              tunnel: w344 -> [w445]
              tunnel: w336 -> [w432]
              frame #0 {
                # "To synch DAQ and scope acquisitions"
                n225 = local read "Averages on scope"() -> (w457:i32)
                n226 = local read "DAQ LED line"() -> (w436:string)
                n227 = Equal?(x=w457, y=1.0) -> (x = y?=w455:bool)
                n228 = call "Initiate.vi"("error in (no error)"=w453, "VISA resource name"=w454) -> ("error out"=w442:errorcluster, "VISA resource name out"=w444:refnum<visa-resource-name>)  [unwired: 8 in]
                n229 = Multiply(x="LED on (s)", y=1000.0) -> (x*y=w437:dbl)
                n230 = case shown="True" w455 {
                  tunnel: [w498 w504] -> w458
                  tunnel: w449 -> [w497 w503]
                  tunnel: w448 -> [w496 w502]
                  tunnel: [w494 w501] -> w447
                  tunnel: [w493 w500] -> w446
                  tunnel: w445 -> [_ w499]
                  frame True {
                    # "No averages on scope, acquire one shot"
                    n231 = call-poly <vilib>:"DAQmx Read.vi"("task/channels in"=w497, "number of samples per channel"=-1, "timeout"=120.0, "error in"=w496) -> ("task out"=w494:refnum<k21>, "data"=w498:waveform(dbl), "error out"=w493:errorcluster)  [unwired: 9 in]
                  }
                  frame False {
                    # "Averaging on scope, acquire multiple shots."
                    n232 = while {
                      shift-right: [w518] -> w504
                      shift-left: w499 -> [w517]
                      tunnel: w503 -> [w511]
                      tunnel: w502 -> [w510]
                      tunnel: [w507] -> w501
                      tunnel: [w506] -> w500
                      i -> [w514]
                      stop <- w516 stop-if-true
                      n233 = call-poly <vilib>:"DAQmx Read.vi"("task/channels in"=w511, "number of samples per channel"=-1, "timeout"=20.0, "error in"=w510) -> ("task out"=w507:refnum<k21>, "data"=w512:waveform(dbl), "error out"=w506:errorcluster)  [unwired: 9 in]
                      n234 = local read "Averages on scope"() -> (w515:i32)
                      n235 = Add(x=w514, y=1) -> (x+y=w508:i32)
                      "DAQ Loop" <- w508
                      n236 = Greater Or Equal?(x=w508, y=w515) -> (x >= y?=w516:bool)
                      n237 = Add(1:w517, 2:w512) -> (0:w518:waveform(dbl))  [unwired: 1 in, 1 out]
                    }
                  }
                }
                n238 = Multiply(x="LED off (s)", y=1000.0) -> (x*y=w433:dbl)
                n239 = case shown="True" "PIA Mode" {
                  tunnel: w444 -> [w460 w474]
                  tunnel: [w460 w468] -> w443
                  tunnel: w442 -> [w459 w473]
                  tunnel: [w459 w469] -> w441
                  tunnel: w437 -> [_ w472]
                  tunnel: w436 -> [_ w467]
                  tunnel: w433 -> [_ w466]
                  tunnel: w432 -> [_ w461]
                  frame False {
                  }
                  frame True {
                    n240 = flat-sequence {
                      tunnel: w467 -> [w483]
                      tunnel: w473 -> [w484]
                      tunnel: w474 -> [w485]
                      tunnel: [w485] -> w465
                      tunnel: [w484] -> w464
                      tunnel: [w483] -> w463
                      tunnel: [w482] -> w462
                      tunnel: w461 -> [w481]
                      tunnel: [w490] -> w471
                      tunnel: [w491] -> w470
                      tunnel: [w489] -> _
                      tunnel: w472 -> [w488]
                      tunnel: w465 -> [w490]
                      tunnel: w464 -> [w491]
                      tunnel: w463 -> [w487]
                      tunnel: w462 -> [_]
                      frame #0 {
                        n241 = Wait (ms)(milliseconds to wait=w481) -> (millisecond timer value=w482:u32)
                      }
                      frame #1 {
                        n242 = call "RG DAQ control for PIA.vi"("lines"=w487, "Initial value"=TRUE) -> ()  [unwired: 10 in]
                        n243 = Wait (ms)(milliseconds to wait=w488) -> (millisecond timer value=w489:u32)
                      }
                    }
                    n244 = flat-sequence {
                      tunnel: w471 -> [w480]
                      tunnel: [w480] -> w468
                      tunnel: [w479] -> _
                      tunnel: w466 -> [w478]
                      tunnel: w467 -> [w477]
                      tunnel: w470 -> [w475]
                      tunnel: [w475] -> w469
                      frame #0 {
                        n245 = call "RG DAQ control for PIA.vi"("lines"=w477, "Initial value"=FALSE) -> ()  [unwired: 10 in]
                        n246 = Wait (ms)(milliseconds to wait=w478) -> (millisecond timer value=w479:u32)
                      }
                    }
                  }
                }
                n247 = VISA Write(VISA resource name=w443, write buffer="*WAI", error in (no error)=w441) -> (VISA resource name out=w451:refnum<visa-resource-name>, error out=w450:errorcluster)  [unwired: 1 out]
              }
            }
            n248 = local read "Scope Timeout (ms)"() -> (w355:u32)
            n249 = local read "DAQ Number of Samples"() -> (w340:dbl)
            n250 = call "RG Fetch Waveforms from scope.vi"("error in (no error)"=w354, "Maximum Time (10000ms)"=w355, "Channels"=w352, "VISA resource name"=w353) -> ("error out"=w349:errorcluster, "Waveform Data"=w351:waveform(dbl)[], "VISA resource name out"=w350:refnum<visa-resource-name>)  [unwired: 5 in]
            n251 = Unbundle By Name(w349) -> ("status"=w361:bool)
            n252 = local read "Scope average\nnumber of points"() -> (w384:dbl)
            n253 = local read "DAQ rate"() -> (w337:i32)
            n254 = Multiply(x=w340, y=-0.1) -> (x*y=w338:dbl)
            n255 = local read "DAQ average number of points"() -> (w375:dbl)
            n256 = Divide(x=w338, y=w337) -> (x/y=w341:dbl)
            n257 = Split Signals(w351) -> (w382:dynamicdata, w381:dynamicdata)  [unwired: 2 in]
            n258 = To Time Stamp(1:w341) -> (0:w342:timestamp)
            n259 = Unbundle By Name(w343) -> ("Y"=w376:dbl[])
            n260 = call "Convert from Dynamic Data2"("Dynamic Data Type"=w382) -> ("Array"=w360:dbl[])  [unwired: 3 in]
            n261 = call "Convert from Dynamic Data3"("Dynamic Data Type"=w381) -> ("Array"=w380:dbl[])  [unwired: 3 in]
            n262 = Empty Array?(array=w360) -> (empty?=w359:bool)
            n263 = Bundle By Name(cluster=w343, "t0"=w342) -> (w329:waveform(dbl))
            n264 = case shown="False" "Inspect Traces" {
              tunnel: [TRUE w392] -> w330
              tunnel: w329 -> [w389 w391]
              frame False {
                n265 = local write "DAQ Live Data"(w389) -> ()
              }
              frame True {
                n266 = call "User trace inspection"() -> ("yes - keep it."=w392:bool)  [unwired: 18 in, 1 out]
                "DAQ Live Data" <- w391
              }
            }
            n267 = call-poly <vilib>:"Decimate (single shot).vi"("averaging"=TRUE, "decimating factor"=w375, "X"=w376) -> ("Decimated Array"=w367:dbl[])  [unwired: 7 in, 1 out]
            n268 = Not Or(1:w359, 2:w361) -> (0:w335:bool)
            n269 = call-poly <vilib>:"Decimate (single shot).vi"("averaging"=TRUE, "decimating factor"=w384, "X"=w360) -> ("Decimated Array"=w372:dbl[])  [unwired: 7 in, 1 out]
            n270 = call-poly <vilib>:"Decimate (single shot).vi"("averaging"=TRUE, "decimating factor"=w384, "X"=w380) -> ("Decimated Array"=w373:dbl[])  [unwired: 7 in, 1 out]
            n271 = Build Array(w328, w330, w328, w335) -> (w334:bool[])
            n272 = Search 1D Array(1D array=w334, element=FALSE) -> (index of element=w332:i32)  [unwired: 1 in]
            n273 = case shown="2, Default" w332 {
              tunnel: [w398 w412 w424] -> w388
              tunnel: [w397 w411 w423] -> w387
              tunnel: [w395 w402 w418] -> w386
              tunnel: w373 -> [_ w410 _]
              tunnel: w372 -> [_ w409 _]
              tunnel: w370 -> [w397 w408 w423]
              tunnel: w369 -> [w395 w407 w418]
              tunnel: w368 -> [w398 w406 w424]
              tunnel: w367 -> [_ w405 _]
              tunnel: [w396 w404 w422] -> w366
              tunnel: w365 -> [w396 w403 w422]
              tunnel: [w395 w402 w418] -> w364
              tunnel: w363 -> [_ _ w420]
              tunnel: w349 -> [w393 w401 w416]
              tunnel: [w393 w401 w414] -> w362
              tunnel: w350 -> [w394 w400 w417]
              tunnel: [w394 w400 w413] -> w358
              frame 1 {
                # "User Rejects Trace"
              }
              frame 2, Default {
                # "No errors"
                n274 = local read "Averages on scope"() -> (w399:i32)
                n275 = Add(x=w399, y=w407) -> (x+y=w402:i32)
                "Readout Counter" <- w402
                n276 = Add(x=w405, y=w406) -> (x+y=w412:dbl[])
                n277 = Add(x=w408, y=w409) -> (x+y=w411:dbl[])
                n278 = Add(x=w410, y=w403) -> (x+y=w404:dbl[])
              }
              frame 3 {
                # "Scope Error Detected"
                n279 = flat-sequence {
                  tunnel: w417 -> [w425]
                  tunnel: w416 -> [w426]
                  tunnel: [w425] -> w415
                  tunnel: w415 -> [w431]
                  tunnel: [w428] -> w414
                  tunnel: [w427] -> w413
                  frame #0 {
                    n280 = call "Close.vi"("error in (no error)"=w426, "VISA resource name"=w425) -> ()  [unwired: 9 in, 1 out]
                  }
                  frame #1 {
                    w430 = FALSE ("ID Query (True)")
                    n281 = call "Initialize.vi"("error in (no error)"=errorcluster {"status"=FALSE, "code"=0, "source"=""}, "Reset (True)"=w430, "ID Query (True)"=w430, "VISA resource name"=w431) -> ("error out"=w428:errorcluster, "VISA resource name out"=w427:refnum<visa-resource-name>)  [unwired: 6 in]
                  }
                }
                n282 = Add(x=w420, y=1.0) -> (x+y=→"Scope Error Counter":dbl)
              }
            }
            n283 = local read "Number of Averages"() -> (w379:i32)
            n284 = Greater Or Equal?(x=w386, y=w379) -> (x >= y?=w378:bool)
            n285 = Or(x=w378, y="Stop Measurement") -> (x .or. y?=w371:bool)
          }
          n286 = call-poly <vilib>:"Index Waveform Array.vi"("index"=0, "waveform array"=w163) -> ("waveform"=w161:waveform(dbl))  [unwired: 8 in, 1 out]
          n287 = Unbundle By Name(w161) -> ("t0"=w141:timestamp, "dt"=w140:dbl)
          n288 = local read "Record Length"() -> (w157:u32)
          n289 = To Double Precision Float(number=w141) -> (double precision float=w160:dbl)
          n290 = Multiply(x=w157, y=1000.0) -> (x*y=w159:dbl)
          n291 = local read "Scope average\nnumber of points"() -> (w154:dbl)
          n292 = for {
            N: w159 -> [_]
            tunnel: w160 -> [w530]
            tunnel: w140 -> [w528]
            tunnel: [w526] -> w156 mode=indexing
            i -> [w529]
            n293 = Multiply(x=w528, y=w529) -> (x*y=w527:dbl)
            n294 = Add(x=w530, y=w527) -> (x+y=w526:dbl)
          }
          n295 = call-poly <vilib>:"Decimate (single shot).vi"("averaging"=TRUE, "decimating factor"=w154, "X"=w156) -> ("Decimated Array"=w153:dbl[])  [unwired: 7 in, 1 out]
          "Scope time axis" <- w153
          n296 = call <vilib>:"DAQmx Clear Task.vi"("task in"=w122, "error in"=w121) -> ()  [unwired: 13 in, 1 out]
          n297 = local read "Averages on scope"() -> (w120:i32)
          n298 = Divide(x=w119, y=w120) -> (x/y=w118:dbl)
          n299 = Divide(x=w264, y=w118) -> (x/y=w306:dbl[])
          n300 = Divide(x=w263, y=w118) -> (x/y=w197:dbl[])
          n301 = local read "DAQ final number of points"() -> (w116:dbl)
          n302 = Bundle By Name("Y"=w306, "t0"=w141, "dt"=w140) -> (→"Scope Average Channel2":waveform(dbl))  [unwired: 1 in]
          n303 = Bundle By Name("Y"=w197, "t0"=w141, "dt"=w140) -> (→"Scope Average Channel1":waveform(dbl))  [unwired: 1 in]
          n304 = local read "DAQ average number of points"() -> (w267:dbl)
          n305 = Divide(x=w297, y=w119) -> (x/y=w164:dbl[])
          n306 = local read "DAQ dt"() -> (w268:dbl)
          n307 = Multiply(x=w116, y=-0.1) -> (x*y=w113:dbl)
          n308 = Multiply(x=w268, y=w267) -> (x*y=w114:dbl)
          n309 = Multiply(x=w113, y=w114) -> (x*y=w111:dbl)
          n310 = To Time Stamp(1:w111) -> (0:w112:timestamp)
          n311 = local read "DAQ final number of points"() -> (w275:dbl)
          n312 = Bundle By Name("Y"=w164, "t0"=w112, "dt"=w114) -> (→"DAQ Average Data":waveform(dbl))  [unwired: 1 in]
          n313 = Multiply(x=w275, y=0.075) -> (x*y=w270:dbl)
          n314 = Round To Nearest(number=w270) -> (nearest integer value=w269:dbl)
          n315 = Array Subset(array=w164, index=0, length=w269) -> (w291:dbl[])
          n316 = local read "Amplification Factor"() -> (w289:dbl)
          n317 = Add Array Elements(numeric array=w291) -> (sum=w290:dbl)
          n318 = Divide(x=w290, y=w269) -> (x/y=w138:dbl)
          n319 = Multiply(x=w138, y=w289) -> (x*y=w139:dbl)
          n320 = local write "Background level (on Amp)"(w139) -> ()
          n321 = local write "Background level (V)"(w138) -> ()
          n322 = local read "DAQ Number of Samples"() -> (w145:dbl)
          n323 = for {
            N: w145 -> [_]
            tunnel: [w520] -> w146 mode=indexing
            i -> [w525]
            n324 = local read "DAQ Number of Samples"() -> (w524:dbl)
            n325 = Divide(x=w524, y=10.0) -> (x/y=w522:dbl)
            n326 = local read "DAQ dt"() -> (w519:dbl)
            n327 = Subtract(x=w525, y=w522) -> (x-y=w521:dbl)
            n328 = Multiply(x=w521, y=w519) -> (x*y=w520:dbl)
          }
          n329 = local read "DAQ average number of points"() -> (w148:dbl)
          n330 = Number To Decimal String(number=w176, width (-)=i16 3) -> (decimal integer string=w175:string)
          n331 = call-poly <vilib>:"Decimate (single shot).vi"("averaging"=TRUE, "decimating factor"=w148, "X"=w146) -> ("Decimated Array"=w144:dbl[])  [unwired: 7 in, 1 out]
          n332 = Concatenate Strings(w175, "nm Scope CH2 (raw data).txt") -> (w189:string)
          n333 = global read "global tas.vi" "Root Path"() -> (w255:path)
          n334 = Build Array(w144, w164) -> (w256:dbl[][])
          n335 = Build Array(w153, w197) -> (w246:dbl[][])
          n336 = global read "global tas.vi" "Root Path"() -> (w250:path)
          n337 = Concatenate Strings(w175, "nm DAQ (raw data).txt") -> (w192:string)
          n338 = global read "global tas.vi" "Root Path"() -> (w174:path)
          n339 = Build Array(w153, w306) -> (w251:dbl[][])
          n340 = Concatenate Strings(w175, "nm Scope CH1 (raw data).txt") -> (w187:string)
          n341 = Build Path(base path=w255, name or relative path=w192) -> (appended path=w254:path)
          n342 = Build Path(base path=w250, name or relative path=w189) -> (appended path=w249:path)
          n343 = Build Path(base path=w174, name or relative path=w187) -> (appended path=w245:path)
          n344 = call-poly <vilib>:"Write To Spreadsheet File.vi"("transpose? (no:F)"=TRUE, "format (%.3f)"="%.9f", "2D data"=w256, "file path (dialog if empty)"=w254) -> ()  [unwired: 4 in, 1 out]
          n345 = call-poly <vilib>:"Write To Spreadsheet File.vi"("transpose? (no:F)"=TRUE, "format (%.3f)"="%.9f", "2D data"=w246, "file path (dialog if empty)"=w245) -> ()  [unwired: 4 in, 1 out]
          n346 = call-poly <vilib>:"Write To Spreadsheet File.vi"("transpose? (no:F)"=TRUE, "format (%.3f)"="%.9f", "2D data"=w251, "file path (dialog if empty)"=w249) -> ()  [unwired: 4 in, 1 out]
          n347 = flat-sequence {
            tunnel: w175 -> [w664]
            tunnel: w174 -> [w663]
            tunnel: w137 -> [_]
            frame #0 {
              # "Write parameters file after values have been calculated."
              n348 = Build Array("Number of Averages", "Scope acq. type", "Number of averages on scope", "Scope average number of points", "Scope timebase (s)", "Scope CH1 vertical scale per div (V)", "Scope CH2 vertical scale per div (V)", "Background level on amp (V)", "DAQ sampling rate (Hz)", "DAQ average number of points", "Background level on DAQ (V)", "Amplification factor", "100% Reflection Reference Signal (V)" ("element"), "Output calculation Method" ("element")) -> (w688:string[])
              n349 = Concatenate Strings(w664, "nm Parameters.txt") -> (w666:string)
              n350 = local read "Averages on scope"() -> (w679:i32)
              n351 = local read "Scope Timebase"() -> (w680:dbl)
              n352 = local read "DAQ rate"() -> (w684:i32)
              n353 = local read "Acquisition Type"() -> (w697:u16)
              n354 = Build Path(base path=w663, name or relative path=w666) -> (appended path=w690:path)
              n355 = local read "Scope average\nnumber of points"() -> (w678:dbl)
              n356 = local read "Vertical Range CH TAS (10.0 V)"() -> (w681:dbl)
              n357 = local read "Vertical Range TPC (10.0 V)"() -> (w682:dbl)
              n358 = local read "Background level (on Amp)"() -> (w683:dbl)
              n359 = local read "DAQ average number of points"() -> (w685:dbl)
              n360 = local read "Background level (V)"() -> (w686:dbl)
              n361 = local read "Amplification Factor"() -> (w687:dbl)
              n362 = local read "100% Reflectance Standard (V)"() -> (w699:dbl)
              n363 = local read "Calculate Output Method"() -> (w701:T1)
              n364 = local read "Readout Counter"() -> (w695:i32)
              n365 = Build Array(w695, w697, w679, w678, w680, w681, w682, w683, w684, w685, w686, w687, w699, w701) -> (w689:dbl[])
              n366 = Number To Fractional String(number=w689) -> (F-format string=w665:string[])  [unwired: 3 in]
              n367 = Build Array(w688, w665) -> (w691:string[][])
              n368 = Array To Spreadsheet String(array=w691, 3:"%s" ("format string")) -> (spreadsheet string=w693:string)  [unwired: 1 in]
              n369 = Write to Text File(file (use dialog)=w690, text=w693) -> ()  [unwired: 2 in, 3 out]
            }
          }
          n370 = local read "Calculate Output Method"() -> (w209:T1)
          n371 = local read "TPC Multiplication factor"() -> (w230:dbl)
          n372 = case shown="\"Kubelka-Munk\"" w209 {
            tunnel: w164 -> [w732 w737 w755]
            tunnel: [w731 w735 w747] -> w229
            tunnel: w138 -> [w730 w734 w738]
            frame "Transmission" {
              # "Background level on DAQ"
              # "Calculate output as: deltaOD = log(T/T')"
              n373 = Divide(x=w730, y=w732) -> (x/y=w733:dbl[])
              n374 = Logarithm Base 10(1:w733) -> (0:w731:dbl[])
            }
            frame "Reflectance" {
              # "Calculate output as: Transient abs. = 1 - RT = (Rbkg - R(t)) / Rbkg"
              n375 = Subtract(x=w734, y=w737) -> (x-y=w736:dbl[])
              n376 = Divide(x=w736, y=w734) -> (x/y=w735:dbl[])
            }
            frame "Kubelka-Munk" {
              # "Calculate output from\nKM = (1-Rrelative)^2/(2*Rrelative)"
              n377 = local read "100% Reflectance Standard (V)"() -> (w754:dbl)
              n378 = Divide(x=w755, y=w754) -> (x/y=w740:dbl[])
              n379 = Subtract(x=1.0, y=w740) -> (x-y=w742:dbl[])
              n380 = Divide(x=w738, y=w754) -> (x/y=w749:dbl)
              n381 = Square(x=w742) -> (x^2=w743:dbl[])
              n382 = Subtract(x=1.0, y=w749) -> (x-y=w752:dbl)
              n383 = Multiply(x=w740, y=2.0) -> (x*y=w744:dbl[])
              n384 = Square(x=w752) -> (x^2=w751:dbl)
              n385 = Divide(x=w743, y=w744) -> (x/y=w739:dbl[])
              n386 = Multiply(x=w749, y=2.0) -> (x*y=w750:dbl)
              n387 = Divide(x=w751, y=w750) -> (x/y=w746:dbl)
              n388 = Subtract(x=w739, y=w746) -> (x-y=w747:dbl[])
            }
          }
          n389 = local read "DAQ average number of points"() -> (w202:dbl)
          n390 = local read "DAQ final number of points"() -> (w213:dbl)
          n391 = Multiply(x=w306, y=w230) -> (x*y=w237:dbl[])
          n392 = local read "DAQ dt"() -> (w203:dbl)
          n393 = local read "Scope pretrigger points"() -> (w217:dbl)
          n394 = Multiply(x=w203, y=w202) -> (x*y=w204:dbl)
          n395 = Divide(x=w213, y=-10.0) -> (x/y=w212:dbl)
          n396 = Multiply(x=w212, y=w204) -> (x*y=w211:dbl)
          n397 = To Time Stamp(1:w211) -> (0:w210:timestamp)
          n398 = Multiply(x=w217, y=0.75) -> (x*y=w216:dbl)
          n399 = Bundle By Name("Y"=w237, "t0"=w141, "dt"=w140) -> (→"Scope CH2 data (final)":waveform(dbl))  [unwired: 1 in]
          n400 = Array Subset(array=w197, index=0, length=w216) -> (w220:dbl[])
          n401 = Add Array Elements(numeric array=w220) -> (sum=w221:dbl)
          n402 = Divide(x=w221, y=w216) -> (x/y=w222:dbl)
          n403 = Subtract(x=w197, y=w222) -> (x-y=w208:dbl[])
          n404 = local read "Calculate Output Method"() -> (w205:T1)
          n405 = Bundle By Name("Y"=w229, "t0"=w210, "dt"=w204) -> (→"DAQ DOD data (final)":waveform(dbl))  [unwired: 1 in]
          n406 = Add(x=w208, y=w139) -> (x+y=w207:dbl[])
          n407 = case shown="\"Reflectance\"" w205 {
            tunnel: w207 -> [w703 w709 w728]
            tunnel: [w702 w706 w721] -> w206
            frame "Transmission" {
              # "Calculate output as: deltaOD = log(T/T')"
              n408 = local read "Background level (on Amp)"() -> (w704:dbl)
              n409 = Divide(x=w704, y=w703) -> (x/y=w705:dbl[])
              n410 = Logarithm Base 10(1:w705) -> (0:w702:dbl[])
            }
            frame "Reflectance" {
              # "Calculate output as: Transient abs. = 1 - RT = (Rbkg - R(t)) / Rbkg"
              n411 = local read "Background level (on Amp)"() -> (w708:dbl)
              n412 = Subtract(x=w708, y=w709) -> (x-y=w707:dbl[])
              n413 = Divide(x=w707, y=w708) -> (x/y=w706:dbl[])
            }
            frame "Kubelka-Munk" {
              # "Calculate output from\nKM = (1-Rrelative)^2/(2*Rrelative)"
              n414 = local read "100% Reflectance Standard (V)"() -> (w711:dbl)
              n415 = local read "Amplification Factor"() -> (w712:dbl)
              n416 = local read "Background level (on Amp)"() -> (w729:dbl)
              n417 = Multiply(x=w711, y=w712) -> (x*y=w710:dbl)
              n418 = Divide(x=w728, y=w710) -> (x/y=w714:dbl[])
              n419 = Subtract(x=1.0, y=w714) -> (x-y=w716:dbl[])
              n420 = Divide(x=w729, y=w710) -> (x/y=w723:dbl)
              n421 = Square(x=w716) -> (x^2=w717:dbl[])
              n422 = Subtract(x=1.0, y=w723) -> (x-y=w726:dbl)
              n423 = Multiply(x=w714, y=2.0) -> (x*y=w718:dbl[])
              n424 = Square(x=w726) -> (x^2=w725:dbl)
              n425 = Divide(x=w717, y=w718) -> (x/y=w713:dbl[])
              n426 = Multiply(x=w723, y=2.0) -> (x*y=w724:dbl)
              n427 = Divide(x=w725, y=w724) -> (x/y=w720:dbl)
              n428 = Subtract(x=w713, y=w720) -> (x-y=w721:dbl[])
            }
          }
          n429 = local read "DAQ Number of Samples"() -> (w218:dbl)
          n430 = for {
            N: w218 -> [_]
            tunnel: [w757] -> w152 mode=indexing
            i -> [w762]
            n431 = local read "DAQ Number of Samples"() -> (w761:dbl)
            n432 = Divide(x=w761, y=10.0) -> (x/y=w759:dbl)
            n433 = local read "DAQ dt"() -> (w756:dbl)
            n434 = Subtract(x=w762, y=w759) -> (x-y=w758:dbl)
            n435 = Multiply(x=w758, y=w756) -> (x*y=w757:dbl)
          }
          n436 = Number To Decimal String(number=w176, width (-)=i16 3) -> (decimal integer string=w178:string)
          n437 = local read "DAQ average number of points"() -> (w149:dbl)
          n438 = Concatenate Strings(w178, "nm Scope CH1 (final A).txt") -> (w180:string)
          n439 = Build Array(w153, w237) -> (w236:dbl[][])
          n440 = global read "global tas.vi" "Root Path"() -> (w226:path)
          n441 = Concatenate Strings(w178, "nm Scope CH2 (final).txt") -> (w182:string)
          n442 = global read "global tas.vi" "Root Path"() -> (w235:path)
          n443 = Build Path(base path=w226, name or relative path=w180) -> (appended path=w225:path)
          n444 = Build Path(base path=w235, name or relative path=w182) -> (appended path=w234:path)
          n445 = call-poly <vilib>:"Decimate (single shot).vi"("averaging"=TRUE, "decimating factor"=w149, "X"=w152) -> ("Decimated Array"=w151:dbl[])  [unwired: 7 in, 1 out]
          n446 = call-poly <vilib>:"Write To Spreadsheet File.vi"("transpose? (no:F)"=TRUE, "format (%.3f)"="%.9f", "2D data"=w236, "file path (dialog if empty)"=w234) -> ()  [unwired: 4 in, 1 out]
          n447 = Bundle By Name("Y"=w206, "t0"=w141, "dt"=w140) -> (w199:waveform(dbl))  [unwired: 1 in]
          "Scope CH1 DOD data (A final)" <- w199
          n448 = Build Array(w151, w229) -> (w228:dbl[][])
          n449 = global read "global tas.vi" "Root Path"() -> (w239:path)
          n450 = Build Array(w153, w206) -> (w227:dbl[][])
          n451 = call-poly <vilib>:"Write To Spreadsheet File.vi"("transpose? (no:F)"=TRUE, "format (%.3f)"="%.9f", "2D data"=w227, "file path (dialog if empty)"=w225) -> ("new file path (Not A Path if cancelled)"=w137:path)  [unwired: 4 in]
          n452 = Concatenate Strings(w178, "nm DAQ DOD (final).txt") -> (w184:string)
          n453 = local read "Trace B ?"() -> (w200:bool)
          n454 = Build Path(base path=w239, name or relative path=w184) -> (appended path=w240:path)
          n455 = case shown="True" w200 {
            tunnel: w199 -> [_ _]
            tunnel: [u32 0 ("millisecond timer value") w886] -> w198
            tunnel: w119 -> [_ _]
            frame False {
            }
            frame True {
              w899 = u32 10000  # timeout (10sec)
              # "Note:Closing the serial port allows it to be used by other applications without quitting LabVIEW."
              # "Close session to port."
              # "Configure Serial port (baud rate, data bits, parity, stop bits and flow control)."
              # "Write bytes to port."
              n456 = Wait (ms)(milliseconds to wait=u32 20000) -> (millisecond timer value=w886:u32)
              n457 = local read "Shutter VISA resource name"() -> (w893:refnum<visa-resource-name>)
              n458 = local read "Shutter data bits"() -> (w890:u16)
              n459 = local read "Shutter baud rate"() -> (w892:u32)
              n460 = local read "Shutter parity"() -> (w891:u16)
              n461 = local read "Shutter flow control"() -> (w889:u16)
              n462 = local read "Shutter stop bits"() -> (w888:u16)
              n463 = local read "Shutter open string"() -> (w885:string)
              n464 = call-poly "VISA Configure Serial Port"("VISA resource name"=w893, "timeout (10sec)"=w899, "baud rate (9600)"=w892, "data bits (8)"=w890, "parity (0:none)"=w891, "stop bits (10: 1 bit)"=w888, "flow control (0:none)"=w889) -> ("VISA resource name out"=w898:refnum<visa-resource-name>, "error out"=w897:errorcluster)  [unwired: 2 in, 5 out]
              n465 = VISA Write(VISA resource name=w898, write buffer=w885, error in (no error)=w897) -> (VISA resource name out=w895:refnum<visa-resource-name>, error out=w894:errorcluster)  [unwired: 1 out]
              n466 = VISA Close(VISA resource name=w895, error in (no error)=w894) -> (error out=w896:errorcluster)
              n467 = call <vilib>:"Simple Error Handler.vi"("error in (no error)"=w896) -> ()  [unwired: 1 in, 8 out]
            }
          }
          n468 = call-poly <vilib>:"Write To Spreadsheet File.vi"("transpose? (no:F)"=TRUE, "format (%.3f)"="%.9f", "2D data"=w228, "file path (dialog if empty)"=w240) -> ()  [unwired: 4 in, 1 out]
          n469 = case shown="True" w200 {
            tunnel: w208 -> [_ w816]
            tunnel: w198 -> [_ _]
            tunnel: [w766 w775] -> w177
            tunnel: w176 -> [_ w774]
            tunnel: w153 -> [_ w773]
            tunnel: w143 -> [w764 w772]
            tunnel: w142 -> [w763 w771]
            frame False {
              n470 = call "Close.vi"("error in (no error)"=w763, "VISA resource name"=w764) -> ("error out"=w765:errorcluster)  [unwired: 9 in]
              n471 = call <vilib>:"Simple Error Handler.vi"("error in (no error)"=w765) -> ()  [unwired: 4 in, 5 out]
              n472 = Wait (ms)(milliseconds to wait=u32 1) -> (millisecond timer value=w766:u32)
            }
            frame True {
              # "Scope time axis"
              # "Current wavelength"
              n473 = local read "Final number of\nscope points"() -> (w788:dbl)
              n474 = Initialize Array(0.0 ("element"), w788) -> (w789:dbl[])
              n475 = while {
                tunnel: w772 -> [w826]
                tunnel: [w835] -> w823
                tunnel: w771 -> [w825]
                tunnel: [w834] -> w824
                shift-right: [w853] -> w791
                shift-left: w789 -> [w852]
                shift-right: [w836] -> w770
                shift-left: 0 -> [w837]
                stop <- w849 stop-if-true
                n476 = local read "Channel TAS (0: Channel 1)"() -> (w831:u16)
                n477 = local read "Scope Timeout (ms)"() -> (w832:u32)
                n478 = call "RG Read (Single Waveform) change OPC for WAIT.vi"("error in (no error)"=w825, "Maximum Time (10000ms)"=w832, "Channel (0: Channel 1)"=w831, "VISA resource name"=w826) -> ("error out"=w828:errorcluster, "Waveform Graph"=w830:waveform(dbl), "VISA resource name out"=w829:refnum<visa-resource-name>)  [unwired: 5 in]
                "B trace (Channel1)" <- w830
                n479 = local read "Scope average\nnumber of points"() -> (w854:dbl)
                n480 = Unbundle By Name(w830) -> ("Y"=w847:dbl[])
                n481 = local read "Final number of\nscope points"() -> (w846:dbl)
                n482 = local read "Averages on scope"() -> (w827:i32)
                n483 = call-poly <vilib>:"Decimate (single shot).vi"("averaging"=TRUE, "decimating factor"=w854, "X"=w847) -> ("Decimated Array"=w843:dbl[])  [unwired: 7 in, 1 out]
                n484 = Array Size(array=w843) -> (size(s)=w842:i32)
                n485 = Initialize Array(0.0 ("element"), w846) -> (w844:dbl[])
                n486 = Equal To 0?(x=w842) -> (x = 0?=w839:bool)
                n487 = Select(t=0.0, s=w839, f=w827) -> (s? t:f=w838:dbl)
                n488 = Add(x=w837, y=w838) -> (x+y=w836:dbl)
                "Btrace Readout Counter" <- w836
                n489 = local read "Number of Averages"() -> (w851:i32)
                n490 = Select(t=w844, s=w839, f=w843) -> (s? t:f=w841:dbl[])
                n491 = VISA Write(VISA resource name=w829, write buffer="*WAI", error in (no error)=w828) -> (VISA resource name out=w835:refnum<visa-resource-name>, error out=w834:errorcluster)  [unwired: 1 out]
                n492 = Add(x=w852, y=w841) -> (x+y=w853:dbl[])
                n493 = Greater Or Equal?(x=w836, y=w851) -> (x >= y?=w850:bool)
                n494 = Or(x=w850, y="Stop Btrace Measurement") -> (x .or. y?=w849:bool)
              }
              n495 = Number To Decimal String(number=w774, width (-)=i16 3) -> (decimal integer string=w777:string)
              n496 = Concatenate Strings(w777, "nm Scope CH1 B trace (raw data).txt") -> (w781:string)
              n497 = global read "global tas.vi" "Root Path"() -> (w793:path)
              n498 = Build Path(base path=w793, name or relative path=w781) -> (appended path=w792:path)
              n499 = local read "Averages on scope"() -> (w769:i32)
              n500 = Divide(x=w770, y=w769) -> (x/y=w768:dbl)
              n501 = local read "Scope pretrigger points"() -> (w800:dbl)
              n502 = Divide(x=w791, y=w768) -> (x/y=w790:dbl[])
              n503 = call "Close.vi"("error in (no error)"=w824, "VISA resource name"=w823) -> ("error out"=w822:errorcluster)  [unwired: 9 in]
              n504 = Build Array(w773, w790) -> (w796:dbl[][])
              n505 = call <vilib>:"Simple Error Handler.vi"("error in (no error)"=w822) -> ()  [unwired: 4 in, 5 out]
              n506 = call-poly <vilib>:"Write To Spreadsheet File.vi"("transpose? (no:F)"=TRUE, "format (%.3f)"="%.9f", "2D data"=w796, "file path (dialog if empty)"=w792) -> ()  [unwired: 4 in, 1 out]
              n507 = Multiply(x=w800, y=0.75) -> (x*y=w801:dbl)
              n508 = Array Subset(array=w790, index=0, length=w801) -> (w819:dbl[])
              n509 = Add Array Elements(numeric array=w819) -> (sum=w820:dbl)
              n510 = Divide(x=w820, y=w801) -> (x/y=w821:dbl)
              n511 = local read "Background level (on Amp)"() -> (w785:dbl)
              n512 = Subtract(x=w790, y=w821) -> (x-y=w817:dbl[])
              n513 = local read "Calculate Output Method"() -> (w797:T1)
              n514 = Subtract(x=w816, y=w817) -> (x-y=w786:dbl[])
              n515 = Add(x=w786, y=w785) -> (x+y=w787:dbl[])
              n516 = case shown="\"Reflectance\"" w797 {
                tunnel: w787 -> [w857 w863 w882]
                tunnel: [w856 w860 w875] -> w798
                frame "Transmission" {
                  # "Calculate output as: deltaOD = log(T/T')"
                  n517 = local read "Background level (on Amp)"() -> (w858:dbl)
                  n518 = Divide(x=w858, y=w857) -> (x/y=w859:dbl[])
                  n519 = Logarithm Base 10(1:w859) -> (0:w856:dbl[])
                }
                frame "Reflectance" {
                  # "Calculate output as: Transient abs. = 1 - RT = (Rbkg - R(t)) / Rbkg"
                  n520 = local read "Background level (on Amp)"() -> (w862:dbl)
                  n521 = Subtract(x=w862, y=w863) -> (x-y=w861:dbl[])
                  n522 = Divide(x=w861, y=w862) -> (x/y=w860:dbl[])
                }
                frame "Kubelka-Munk" {
                  # "Calculate output from\nKM = (1-Rrelative)^2/(2*Rrelative)"
                  n523 = local read "100% Reflectance Standard (V)"() -> (w865:dbl)
                  n524 = local read "Amplification Factor"() -> (w866:dbl)
                  n525 = local read "Background level (on Amp)"() -> (w883:dbl)
                  n526 = Multiply(x=w865, y=w866) -> (x*y=w864:dbl)
                  n527 = Divide(x=w882, y=w864) -> (x/y=w868:dbl[])
                  n528 = Subtract(x=1.0, y=w868) -> (x-y=w870:dbl[])
                  n529 = Divide(x=w883, y=w864) -> (x/y=w877:dbl)
                  n530 = Square(x=w870) -> (x^2=w871:dbl[])
                  n531 = Subtract(x=1.0, y=w877) -> (x-y=w880:dbl)
                  n532 = Multiply(x=w868, y=2.0) -> (x*y=w872:dbl[])
                  n533 = Square(x=w880) -> (x^2=w879:dbl)
                  n534 = Divide(x=w871, y=w872) -> (x/y=w867:dbl[])
                  n535 = Multiply(x=w877, y=2.0) -> (x*y=w878:dbl)
                  n536 = Divide(x=w879, y=w878) -> (x/y=w874:dbl)
                  n537 = Subtract(x=w867, y=w874) -> (x-y=w875:dbl[])
                }
              }
              n538 = local read "Scope pretrigger points"() -> (w802:dbl)
              n539 = local read "Scope Timebase"() -> (w803:dbl)
              n540 = Divide(x=w803, y=10.0) -> (x/y=w809:dbl)
              n541 = Divide(x=w803, y=w802) -> (x/y=w804:dbl)
              n542 = Multiply(x=w809, y=-1.0) -> (x*y=w806:dbl)
              n543 = To Time Stamp(1:w806) -> (0:w805:timestamp)
              n544 = global read "global tas.vi" "Root Path"() -> (w811:path)
              n545 = Bundle By Name("Y"=w798, "t0"=w805, "dt"=w804) -> (→"Scope CH1 DOD data (A-B final)":waveform(dbl))  [unwired: 1 in]
              n546 = Concatenate Strings(w777, "nm Scope CH1 (final A-B).txt") -> (w779:string)
              n547 = Build Path(base path=w811, name or relative path=w779) -> (appended path=w812:path)
              n548 = Wait (ms)(milliseconds to wait=u32 1) -> (millisecond timer value=w775:u32)
              n549 = Build Array(w773, w798) -> (w810:dbl[][])
              n550 = call-poly <vilib>:"Write To Spreadsheet File.vi"("transpose? (no:F)"=TRUE, "format (%.3f)"="%.9f", "2D data"=w810, "file path (dialog if empty)"=w812) -> ()  [unwired: 4 in, 1 out]
            }
          }
        }
        n551 = flat-sequence {
          tunnel: w61 -> [_]
          frame #0 {
            w94 = FALSE
            n552 = local write "2b - Spectrum"(w94) -> ()
            n553 = local write "2a - Kinetic"(w94) -> ()
            n554 = One Button Dialog(message="Acquisition complete.") -> ()  [unwired: 1 in, 1 out]
          }
        }
      }
      frame 3 {
        # "Code"
        n555 = case shown="False" w982 {
          tunnel: w982 -> [w1059 w1073]
          tunnel: [w1056 w1073] -> w981
          frame False {
            # "PTI Mono"
            n556 = flat-sequence {
              tunnel: [w1066] -> w1060
              tunnel: w1059 -> [w1066]
              tunnel: w1060 -> [w1072]
              tunnel: [w1072] -> w1057
              tunnel: [w1068] -> w1058
              frame #0 {
                # "Check where mono is"
                n557 = call "UserInputMonoValue.vi"() -> ("Monochromator readout"=w1067:dbl)  [unwired: 17 in, 2 out]
                n558 = local write "Current Wavelength (PTI)"(w1067) -> ()
              }
              frame #1 {
                # "Find out which grating is currently being used"
                n559 = Two Button Dialog(message="Please press the appropriate\nbutton for the grating currently\nselected on the monochromator.", 1:"Visible" ("F button name (\"Cancel\")"), 2:"IR" ("T button name (\"OK\")")) -> (T button?=w1068:bool)
                n560 = local write "Is IR"(w1068) -> ()
              }
            }
            n561 = case shown="True" w1058 {
              tunnel: w1057 -> [w1061 w1062]
              tunnel: [w1061 w1062] -> w1056
              frame False {
              }
              frame True {
                n562 = local read "Current Wavelength (PTI)"() -> (w1065:dbl)
                n563 = Multiply(x=w1065, y=2.0) -> (x*y=w1064:dbl)
                n564 = local write "Current Wavelength (PTI)"(w1064) -> ()
              }
            }
          }
          frame True {
            # "Oriel Mono"
          }
        }
        n565 = case shown="True" w981 {
          tunnel: [w984 w1044] -> w983
          frame False {
            # "PTI Mono"
            n566 = flat-sequence {
              tunnel: [w988] -> w985
              tunnel: [w1038] -> _
              tunnel: w985 -> [w1038]
              tunnel: [w1037] -> w984
              frame #0 {
                n567 = local read "Is IR"() -> (w987:bool)
                n568 = call "RG Get User Input Wavelength.vi"() -> ("Go to wavelength"=w986:i32)  [unwired: 11 in]
                n569 = case shown="True" w987 {
                  tunnel: [w991 w1014] -> w988
                  tunnel: w986 -> [w990 w1013]
                  tunnel: w986 -> [w989 w1012]
                  frame True {
                    # "Currently in IR"
                    n570 = Greater?(x=w989, y=1000.0) -> (0:w992:bool)
                    n571 = case shown="True" w992 {
                      tunnel: [w995 w1004] -> w991
                      tunnel: w990 -> [w994 w1003]
                      frame False {
                        n572 = stacked-sequence {
                          seq-local: [_ w1000 _] -> [_ _ w1002]
                          tunnel: [_ _ w1002] -> w995
                          tunnel: w994 -> [_ w1000 _]
                          frame #0 {
                            # "switch to visible\nand recal mono"
                            n573 = One Button Dialog(message="Please switch\nto the visible grating\nnow.") -> (true=w996:bool)  [unwired: 1 in]
                            n574 = case shown="True" w996 {
                              frame False {
                              }
                              frame True {
                                n575 = call "UserInputMonoValue.vi"() -> ("Monochromator readout"=w998:dbl)  [unwired: 17 in, 2 out]
                                n576 = local write "Is IR"(FALSE ("Is IR")) -> ()
                                n577 = local write "Current Wavelength (PTI)"(w998) -> ()
                              }
                            }
                          }
                          frame #1 {
                            # "now in visible, move \nto new wavelength"
                            n578 = local read "Current Wavelength (PTI)"() -> (w1001:dbl)
                            n579 = call "ChazMoveMono.vi"("Move to"=w1000, "Current"=w1001) -> ()  [unwired: 8 in, 2 out]
                          }
                          frame #2 {
                            n580 = local write "Current Wavelength (PTI)"(w1002) -> ()
                          }
                        }
                      }
                      frame True {
                        # "Still in IR"
                        n581 = stacked-sequence {
                          seq-local: [w1005 _] -> [_ w1011]
                          tunnel: [_ w1011] -> w1004
                          tunnel: w1003 -> [w1005 _]
                          frame #0 {
                            n582 = local read "Current Wavelength (PTI)"() -> (w1010:dbl)
                            n583 = Divide(x=w1005, y=2.0) -> (x/y=w1006:dbl)
                            n584 = Divide(x=w1010, y=2.0) -> (x/y=w1007:dbl)
                            n585 = call "ChazMoveMono.vi"("Move to"=w1006, "Current"=w1007) -> ()  [unwired: 8 in, 2 out]
                          }
                          frame #1 {
                            n586 = local write "Current Wavelength (PTI)"(w1011) -> ()
                          }
                        }
                      }
                    }
                  }
                  frame False {
                    # "Currently in Visible"
                    n587 = Greater?(x=w1012, y=1000.0) -> (0:w1015:bool)
                    n588 = case shown="True" w1015 {
                      tunnel: [w1018 w1023] -> w1014
                      tunnel: w1013 -> [w1017 w1022]
                      frame False {
                        # "Still in Visible"
                        n589 = stacked-sequence {
                          seq-local: [w1019 _] -> [_ w1021]
                          tunnel: [_ w1021] -> w1018
                          tunnel: w1017 -> [w1019 _]
                          frame #0 {
                            n590 = local read "Current Wavelength (PTI)"() -> (w1020:dbl)
                            n591 = call "ChazMoveMono.vi"("Move to"=w1019, "Current"=w1020) -> ()  [unwired: 8 in, 2 out]
                          }
                          frame #1 {
                            n592 = local write "Current Wavelength (PTI)"(w1021) -> ()
                          }
                        }
                      }
                      frame True {
                        n593 = stacked-sequence {
                          seq-local: [_ w1030 _] -> [_ _ w1036]
                          tunnel: [_ _ w1036] -> w1023
                          tunnel: w1022 -> [_ w1030 _]
                          frame #0 {
                            # "switch to IR\nand recal mono"
                            n594 = One Button Dialog(message="Please switch\nto the IR grating\nnow.") -> (true=w1024:bool)  [unwired: 1 in]
                            n595 = case shown="True" w1024 {
                              frame False {
                              }
                              frame True {
                                n596 = call "UserInputMonoValue.vi"() -> ("Monochromator readout"=w1028:dbl)  [unwired: 17 in, 2 out]
                                n597 = local write "Is IR"(TRUE ("Is IR")) -> ()
                                n598 = Multiply(x=w1028, y=2.0) -> (x*y=w1026:dbl)
                                n599 = local write "Current Wavelength (PTI)"(w1026) -> ()
                              }
                            }
                          }
                          frame #1 {
                            # "now in IR, move \nto new wavelength"
                            n600 = local read "Current Wavelength (PTI)"() -> (w1033:dbl)
                            n601 = Divide(x=w1030, y=2.0) -> (x/y=w1031:dbl)
                            n602 = Divide(x=w1033, y=2.0) -> (x/y=w1032:dbl)
                            n603 = call "ChazMoveMono.vi"("Move to"=w1031, "Current"=w1032) -> ()  [unwired: 8 in, 2 out]
                          }
                          frame #2 {
                            n604 = local write "Current Wavelength (PTI)"(w1036) -> ()
                          }
                        }
                      }
                    }
                  }
                }
              }
              frame #1 {
                n605 = call <vilib>:"General Error Handler.vi"() -> ("error out"=w1037:errorcluster)  [unwired: 11 in, 4 out]
              }
            }
          }
          frame True {
            # "Oriel Mono"
            n606 = call "m_open.vi"() -> ("error out"=w1054:errorcluster, "configuration file path copy"=w1055:path)  [unwired: 2 in]
            n607 = call "GetWave.vi"("error in (no error)"=w1054) -> ("error out"=w1047:errorcluster, "Present Wavelength"=w1043:dbl)  [unwired: 1 in]
            n608 = call "RG Get User Input Wavelength.vi"("Current wavelength"=w1043) -> ("Go to wavelength"=w1042:i32)  [unwired: 10 in]
            n609 = call "getgrat.vi"("error in (no error)"=w1047) -> ("error out"=w1048:errorcluster, "Grating"=→"Grating":i32)  [unwired: 1 in]
            n610 = Less Or Equal?(x=w1042, y=590.0) -> (x <= y?=w1045:bool)
            n611 = Select(t=1.0, s=w1045, f=2.0) -> (s? t:f=w1049:dbl)
            n612 = call "setgrat.vi"("error in (no error)"=w1048, "Grating"=w1049) -> ("error out"=w1046:errorcluster)  [unwired: 1 in]
            n613 = call "gowave.vi"("error in (no error)"=w1046, "Destination Wavelength"=w1042) -> ("error out"=w1041:errorcluster)
            n614 = call "GetWave.vi"("error in (no error)"=w1041) -> ("error out"=w1040:errorcluster, "Present Wavelength"=w1039:dbl)  [unwired: 1 in]
            n615 = local write "Current wavelength (Oriel)"(w1039) -> ()
            n616 = call "m_close.vi"("error in (no error)"=w1040, "configuration file path"=w1055) -> ("error out"=w1044:errorcluster)  [unwired: 1 out]
          }
        }
        n617 = flat-sequence {
          tunnel: w983 -> [_]
          frame #0 {
            n618 = local write "3 - Move mono"(FALSE ("3 - Move shutter")) -> ()
            n619 = One Button Dialog(message="Wavelength change complete.") -> ()  [unwired: 1 in, 1 out]
          }
        }
      }
    }
  }
